vi "RT.vi"() -> ()   [LabVIEW 2012]
uses:
  Type/_RT Instrument State.ctl
  Type/RT Loop Events.ctl
  Type/_RT Parameter.ctl
  Type/_RT Active Ch.ctl
  Type/_RT Expt.ctl
  Type/_Run Mode.ctl
  Type/_RT Mass Range.ctl
  Type/_RT Res Type.ctl
  Type/_LED States.ctl
  Type/_LCD Line1 Msg.ctl
  Type/_LCD Line2 Msg.ctl
  Type/_RT LED Num.ctl
  Type/_Pump Parameter.ctl
  Type/_RW Status.ctl
  Type/_RT Serial Command.ctl
  Type/_FPGA Indicator.ctl
  _RT Global.vi
  <vilib>/FPGAPlugInAG/sbRIO-9602/niLvFpga_Open_sbRIO-9602.vi
  <vilib>/Utility/error.llb/Error Cluster From Error Code.vi
  <vilib>/rvi/errors/niLvFpgaAdjustHostInterfaceError.vi
  <vilib>/Utility/config.llb/Read Key (Boolean).vi
  <vilib>/Utility/config.llb/Read Key (String).vi
  <vilib>/Utility/config.llb/Write Key (Boolean).vi
  <vilib>/Utility/config.llb/Write Key (String).vi
  <vilib>/rvi/interface/nirviOpenFPGA/nirviOpenFPGA.xnode
  FPGA Bitfiles/FPGA9602.lvbitx
  <vilib>/rvi/interface/nirviMethod/nirviMethod.xnode
  <vilib>/rvi/interface/nirviReadWriteControl/nirviReadWriteControl.xnode
  <vilib>/Utility/config.llb/NI_LVConfig.lvlib
  <vilib>/NI_Real-Time Target Support.lvlib
  <vilib>/rvi/errors/niLvFpgaMergeErrorWithErrorCode.vi
  NiFpgaLv.dll
  <vilib>/FPGAPlugInAG/sbRIO-9602/niLvFpga_ConfigureFifo_sbRIO-9602.vi
  <vilib>/FPGAPlugInAG/sbRIO-9602/niLvFpga_StartFifo_sbRIO-9602.vi
panel:
  out "Disconnection#":u8
  out "Message Type":string
  out "Rt Loop Events":T1
  out "code":i32
  out "InstrState":T2=enum."Mass Spectrometer is Off"
  out "Fault":bool
  out "Ready":bool
  out "Running":bool
  out "RunMode":i32
  in  "RT Version":u32=900140920
  out "FPGA Version":u32
  out "Time (s)":dbl
  out "Connected?":bool
  # "Run  Status"
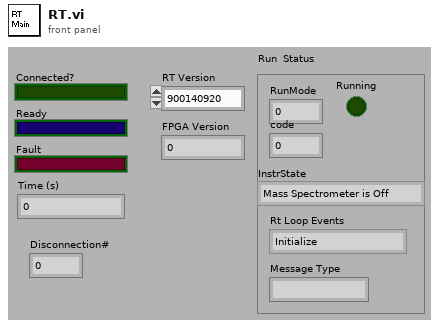
[diagram p1: front panel]
types:
  T1 = typedef "RT Loop Events.ctl" = enum16{"Initialize", "Wait for Connection", "Wait for Command", "Send Reply"}
  T2 = typedef "_RT Instrument State.ctl" = enum16{"Initializing", "Mass Spectrometer is Off", "Starting Up", "Turning Power Off", "Going to Standby", "Roughing Pump Ready", "Turning Turbo Off", "Turbo Startup", "Turbopump Ready", "Checking Vacuum", "Going to Ready", "Ready", "Running", "Source Standby", "Lost Communication", "Shutting Down", "Fault", "24V Standby", "Go to 24V Standby", "Turbopump Ready-Waiting"}
  T3 = typedef "_RT Parameter.ctl" = cluster{"RunMode":i32, "Initial Ch":T4[], "Sync":u8, "Expt":T5[], "EqTime(mS)":i32}
  T4 = typedef "_RT Active Ch.ctl" = cluster{"Start":i32, "Step":i32, "ChID":i32}
  T5 = typedef "_RT Expt.ctl" = cluster{"StartT(mS)":i32, "#Cycles":i32, "Scan Type":T6, "PauseT(uS)":i32, "Polarity":u8, "DelayT(mS)":i32, "Active Ch":T4[], "Mass Range":T7[]}
  T6 = typedef "_Run Mode.ctl" = enum16{"MRM (Q1/Q2)", "Q1 Scan", "Q1 SRM", "Q2 Scan", "Q2 SRM", "Product Scan", "Precursor Scan", "Neutral Loss", "Neutral Gain"}
  T7 = typedef "_RT Mass Range.ctl" = cluster{"Steps":i32, "Dwell(uS)":i32, "Resolution Type":T8, "Ramping Ch":T4[]}
  T8 = typedef "_RT Res Type.ctl" = u16
  T9 = typedef "Semaphore RefNum" = refnum<k1>
  T10 = typedef "_RT Instrument 2.ctl" = cluster{"Table":T11[], "Instrument":string[]}
  T11 = typedef "_RT Configuration 2.ctl" = cluster{"Name":string, "Ch#":u8, "Min":dbl, "Max":dbl, "Def+":dbl, "Def-":dbl, "Offset":dbl, "Slope":dbl, "Type":u8, "Description":string, "SettleT":dbl}
  T12 = cluster{"Rt Loop Events":T1, "Connection ID":refnum<k5>, "Parameter":T3, "Info":string, "Data Array":i32[], "error":errorcluster}
  T13 = typedef "_Pump Parameter.ctl" = enum16{"Turn Pump Motor On", "Turn Pump Motor Off", "Read Pump Oil Deficiency", "Read Rotation Switch Point Attained", "Read Ele. Drive Over Temperature", "Read Pump Over Temperature", "Read Set Rotation Speed Attained", "Read Turbopump Accelerates", "Read Actual Rotation Speed in Hz", "Read Motor Current in A", "Read Operating Hours in h", "Read Motor Voltage in V", "Read Motor Power in W", "Set Rotation Speed Switchpoint in %", "Clear Error", "Read Error Code", "Read Bearing Temperature", "Read Hardware Version", "Read Firmware Version", "Read Operating Hours (Drive)", "Read Rotational Speed (rpm)", "Read Power Stage Temperature", "Read Electronics Temperature", "Read Upper Pump Temperature", "Read Motor Temperature", "Read Error Code History, 1", "Read Error Code History, 2", "Read Error Code History, 3", "Read Error Code History, 4", "Read Error Code History, 5", "Read Error Code History, 6", "Read Error Code History, 7", "Read Error Code History, 8", "Read Error Code History, 9", "Read Error Code History, 10"}
  T14 = typedef "_RW Status.ctl" = enum8{"Done", "Do Read", "Do Write", "Set Latch1", "Set Latch2", "Set Latch3", "Set Latch4", "RP ON", "EL ON", "Serial Send", "Set LC Out", "Get LC In", "Read VAC", "Table Test", "Get Interlock", "Do Read2", "Do Write2"}
  T15 = typedef "_RT Serial Command.ctl" = cluster{"Port Type":u16, "baud rate (9600)":u32, "data bits (8)":u16, "stop bits (1)":u16, "parity (0:none)":u16, "DoRead":bool, "Command":string}
  T16 = typedef "_FPGA Indicator.ctl" = enum16{"Done", "Ready", "Count Available", "SendSerial", "LED State"}
  T17 = typedef "NI_LVConfig.lvlib/Config Data RefNum.ctl" = refnum<k1>
  T18 = typedef "_RT Startup Options.ctl" = cluster{"Door":bool, "Curtain":bool, "Pressure":bool, "Turbo":bool, "SysPoll":bool, "GasFlag":bool}
  T19 = cluster{"Info":string, "Data Array":i32[], "error":errorcluster}
  T20 = typedef "_RT LED Num.ctl" = enum8{"ReadKey", "ClearKeyBuffer", "ClearLCD", "BacklightOn"}
  T21 = typedef "_LED States.ctl" = enum8{"Idle", "Solid B", "Solid R", "Solid P", "Off B", "Off R", "Off P", "Off BRP", "Off RP", "Flash R&P", "Flash P"}
  T22 = typedef "_LCD Line2 Msg.ctl" = u16
  T23 = typedef "_LCD Line1 Msg.ctl" = u16
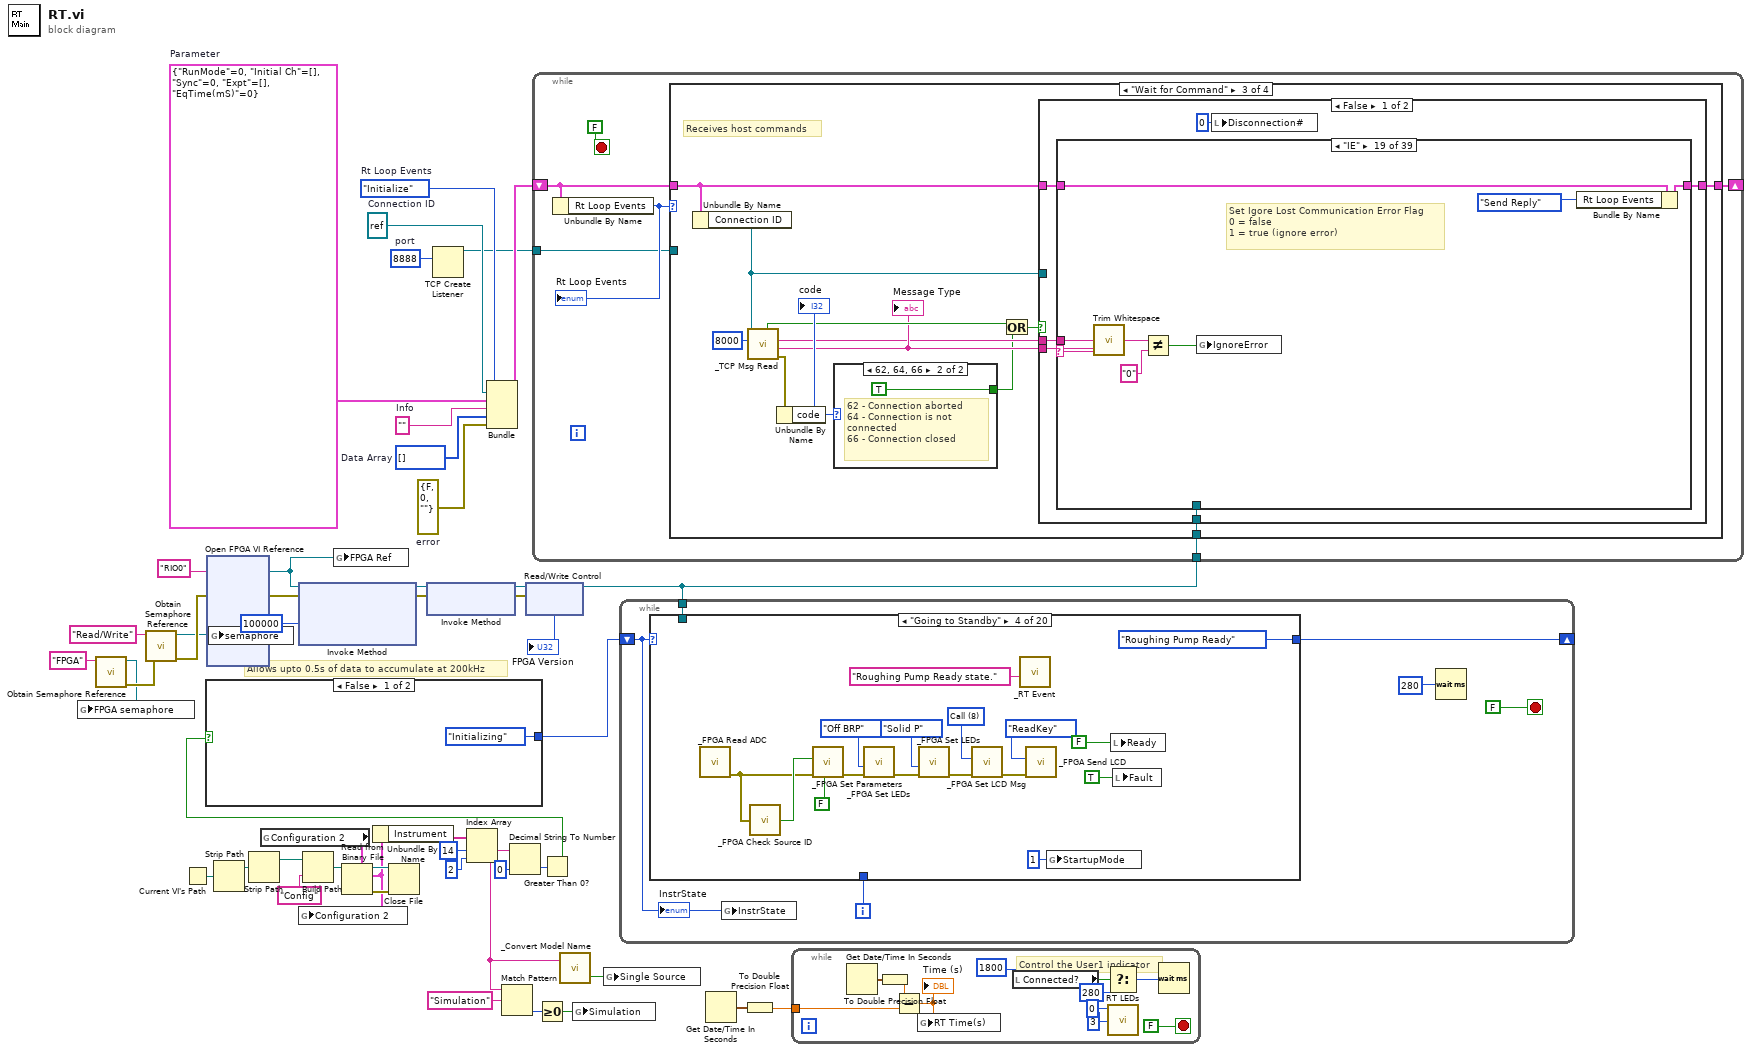
[diagram p0: block diagram]
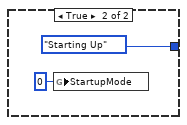
[diagram p2: hidden frame]
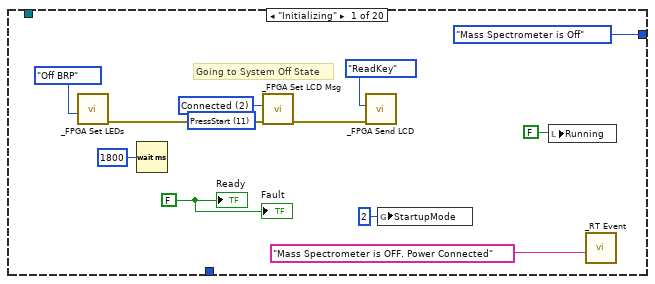
[diagram p3: hidden frame]
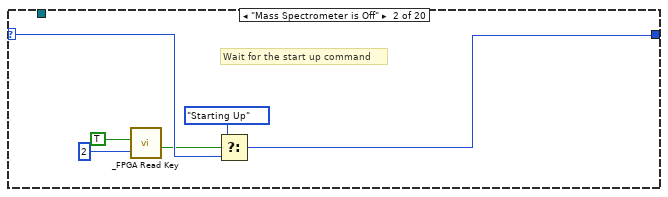
[diagram p4: hidden frame]
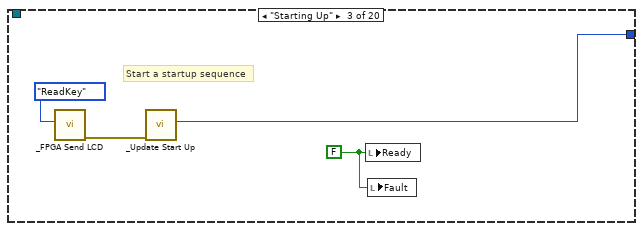
[diagram p5: hidden frame]
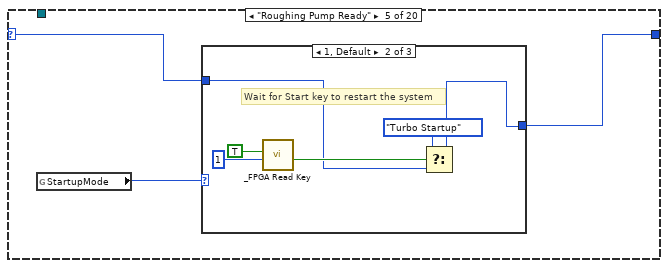
[diagram p6: hidden frame]
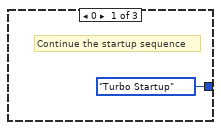
[diagram p7: hidden frame]
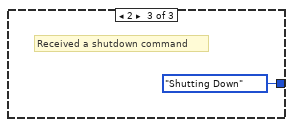
[diagram p8: hidden frame]
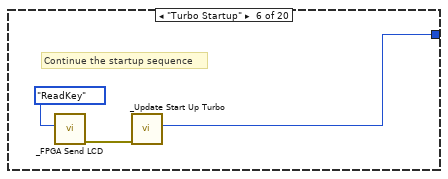
[diagram p9: hidden frame]
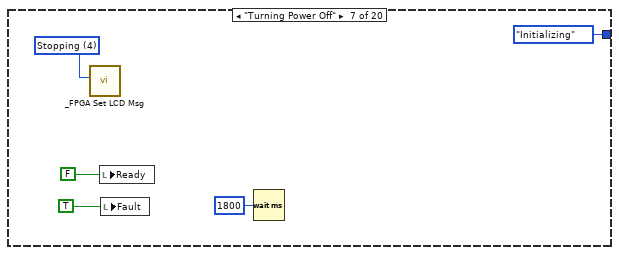
[diagram p10: hidden frame]
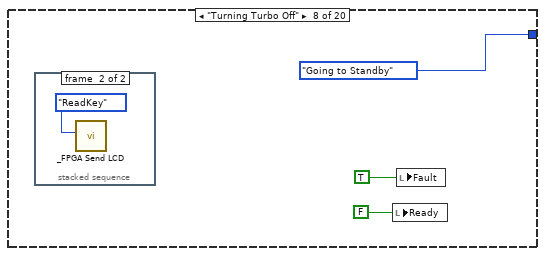
[diagram p11: hidden frame]
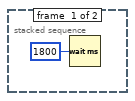
[diagram p12: hidden frame]
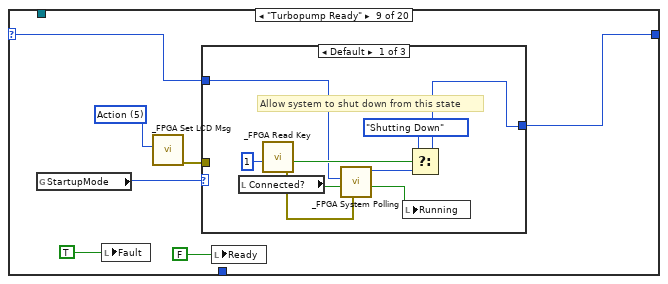
[diagram p13: hidden frame]
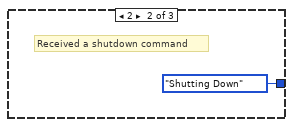
[diagram p14: hidden frame]
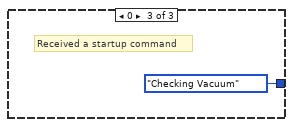
[diagram p15: hidden frame]
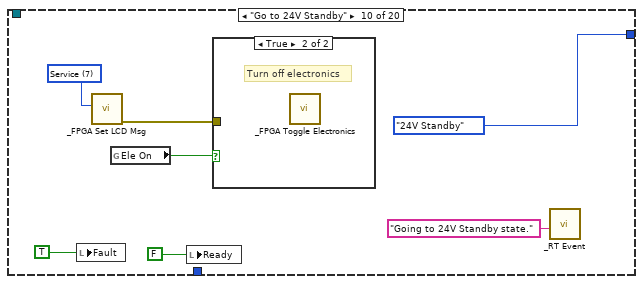
[diagram p16: hidden frame]
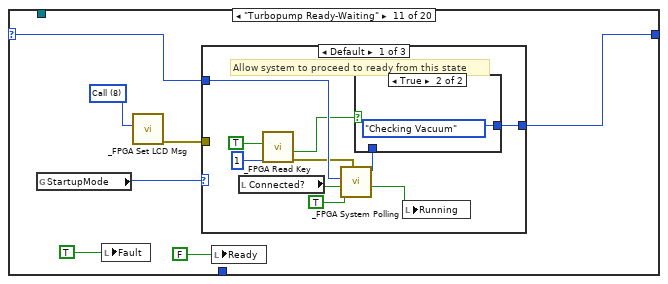
[diagram p18: hidden frame]
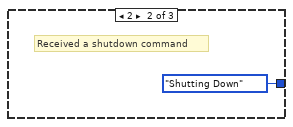
[diagram p20: hidden frame]
diagram:
  w34 = T3 {"RunMode"=0, "Initial Ch"=[], "Sync"=0, "Expt"=[], "EqTime(mS)"=0}  # Parameter
  w36 = u16 8888  # port
  w44 = i32[] []  # Data Array
  w45 = ""  # Info
  w46 = errorcluster {"status"=FALSE, "code"=0, "source"=""}  # error
  w48 = refnum<k5> refnum  # Connection ID
  w49 = RT_Loop_Events."Initialize"  # Rt Loop Events
  # "Allows upto 0.5s of data to accumulate at 200kHz"
  n1 = call <vilib>:"Obtain Semaphore Reference.vi"("name (unnamed)"="FPGA") -> ("error out"=w13:errorcluster, "semaphore"=w11:T9)  [unwired: 2 in, 3 out]
  n2 = global write "_RT Global.vi" "FPGA semaphore"(w11) -> ()
  n3 = call <vilib>:"Obtain Semaphore Reference.vi"("error in (no error)"=w13, "name (unnamed)"="Read/Write") -> ("error out"=w16:errorcluster, "semaphore"=w15:T9)  [unwired: 1 in, 3 out]
  n4 = Current VI's Path() -> (path=w31:path)
  n5 = xnode "Open FPGA VI Reference"("error in"=w16, "resource name"="RIO0") -> ("FPGA VI Reference Out"=w1:refnum<k20>, "error out"=w38:errorcluster)
  n6 = global write "_RT Global.vi" "semaphore"(w15) -> ()
  n7 = Strip Path(path=w31) -> (stripped path=w32:path)  [unwired: 1 out]
  n8 = Strip Path(path=w32) -> (stripped path=w25:path)  [unwired: 1 out]
  n9 = global read "_RT Global.vi" "Configuration 2"() -> (w28:T10)
  n10 = xnode "Invoke Method"("FPGA VI Reference In"=w1, "error in"=w38, "Requested Depth"=u32 100000 ("Depth")) -> ("FPGA VI Reference Out"=w40:refnum<k20>, "error out"=w41:errorcluster)  [unwired: 1 out]
  n11 = Build Path(base path=w25, name or relative path="Config" ("key")) -> (appended path=w30:path)
  n12 = global write "_RT Global.vi" "FPGA Ref"(w1) -> ()
  n13 = Read from Binary File(5:w28, 11:w30) -> (0:w27:errorcluster, 2:w24:T10, 3:w26:refnum<file>)  [unwired: 1 in, 4 out]
  n14 = global write "_RT Global.vi" "Configuration 2"(w24) -> ()
  n15 = Unbundle By Name(w24) -> ("Instrument"=w23:string[])
  n16 = Close File(refnum=w26, error in=w27) -> ()  [unwired: 2 out]
  n17 = xnode "Invoke Method"("FPGA VI Reference In"=w40, "error in"=w41) -> ("FPGA VI Reference Out"=w42:refnum<k20>, "error out"=w43:errorcluster)
  n18 = TCP Create Listener(10:w36) -> (3:w35:refnum<k5>)  [unwired: 1 in, 5 out]
  n19 = Index Array(array=w23, index #1=14 ("index"), index #2=2 ("index")) -> (element #1=w20:string, element #2=w6:string)
  n20 = Bundle("Rt Loop Events"=w49, "Connection ID"=w48, "Parameter"=w34, "Info"=w45, "Data Array"=w44, "error"=w46) -> (w47:T12)  [unwired: 1 out]
  n21 = Match Pattern(string=w6, regular expression="Simulation") -> (offset past match=w9:i32)  [unwired: 4 out]
  n22 = Decimal String To Number(string=w20, default (0L)=0 ("default (0 I32)")) -> (number=w19:i32)  [unwired: 2 out]
  n23 = xnode "Read/Write Control"("FPGA VI Reference In"=w42, "error in"=w43) -> ("FPGA VI Reference Out"=w4:refnum<k20>, "Version"=→"FPGA Version":u32)  [unwired: 1 out]
  n24 = while {
    shift-right: [w52] -> _
    shift-left: w47 -> [w53]
    tunnel: w4 -> [w51]
    tunnel: w35 -> [w50]
    stop <- FALSE stop-if-true
    n25 = Unbundle By Name(w53) -> ("Rt Loop Events"=w54:T1)
    "Rt Loop Events" <- w54
    n26 = case shown="\"Wait for Command\"" w54 {
      tunnel: w53 -> [w83 w124 w144 w782]
      tunnel: [w82 w123 w143 w781] -> w52
      tunnel: w51 -> [_ _ w139 _]
      tunnel: w50 -> [_ w121 _ _]
      frame "Initialize", Default {
        w56 = FALSE ("Connected?")
        w76 = FALSE ("Connected?")
        w69 = "RT" ("section")
        # "Initialize All Instrument Parameters"
        n27 = stacked-sequence {
          frame #0 {
            n28 = call "_Read RT Table.vi"("key"="Cal") -> ("Table"=w85:dbl[][])  [unwired: 2 in, 4 out]
            n29 = global write "_RT Global.vi" "Q1 Cal"(w85) -> ()
            n30 = call "_Read RT Table.vi"("key"="Cal2") -> ("Table"=w86:dbl[][])  [unwired: 2 in, 4 out]
            n31 = global write "_RT Global.vi" "Q2 Cal"(w86) -> ()
            n32 = call "_Read RT Table.vi"("key"="Cal3") -> ("Table"=w87:dbl[][])  [unwired: 2 in, 4 out]
            n33 = global write "_RT Global.vi" "Q1 -Cal"(w87) -> ()
            n34 = call "_Read RT Table.vi"("key"="Cal4") -> ("Table"=w88:dbl[][])  [unwired: 2 in, 4 out]
            n35 = global write "_RT Global.vi" "Q2 -Cal"(w88) -> ()
            n36 = call "_Read RT Table.vi"("key"="Res") -> ("Table"=w89:dbl[][])  [unwired: 2 in, 4 out]
            n37 = global write "_RT Global.vi" "Q1 Res Hi"(w89) -> ()
            n38 = call "_Read RT Table.vi"("key"="Res2") -> ("Table"=w90:dbl[][])  [unwired: 2 in, 4 out]
            n39 = global write "_RT Global.vi" "Q2 Res Hi"(w90) -> ()
            n40 = call "_Read RT Table.vi"("key"="Res3") -> ("Table"=w91:dbl[][])  [unwired: 2 in, 4 out]
            n41 = global write "_RT Global.vi" "Q1 Res Med"(w91) -> ()
            n42 = call "_Read RT Table.vi"("key"="Res4") -> ("Table"=w92:dbl[][])  [unwired: 2 in, 4 out]
            n43 = global write "_RT Global.vi" "Q2 Res Med"(w92) -> ()
            n44 = call "_Read RT Table.vi"("key"="Res5") -> ("Table"=w93:dbl[][])  [unwired: 2 in, 4 out]
            n45 = global write "_RT Global.vi" "Q1 Res Lo"(w93) -> ()
            n46 = call "_Read RT Table.vi"("key"="Res6") -> ("Table"=w94:dbl[][])  [unwired: 2 in, 4 out]
            n47 = global write "_RT Global.vi" "Q2 Res Lo"(w94) -> ()
            n48 = call "_Read RT Table.vi"("key"="Res7") -> ("Table"=w95:dbl[][])  [unwired: 2 in, 4 out]
            n49 = global write "_RT Global.vi" "Q1 -Res Hi"(w95) -> ()
            n50 = call "_Read RT Table.vi"("key"="Res8") -> ("Table"=w96:dbl[][])  [unwired: 2 in, 4 out]
            n51 = global write "_RT Global.vi" "Q2 -Res Hi"(w96) -> ()
            n52 = call "_Read RT Table.vi"("key"="Res9") -> ("Table"=w97:dbl[][])  [unwired: 2 in, 4 out]
            n53 = global write "_RT Global.vi" "Q1 -Res Med"(w97) -> ()
            n54 = call "_Read RT Table.vi"("key"="Res10") -> ("Table"=w98:dbl[][])  [unwired: 2 in, 4 out]
            n55 = global write "_RT Global.vi" "Q2 -Res Med"(w98) -> ()
            n56 = call "_Read RT Table.vi"("key"="Res11") -> ("Table"=w99:dbl[][])  [unwired: 2 in, 4 out]
            n57 = global write "_RT Global.vi" "Q1 -Res Lo"(w99) -> ()
            n58 = call "_Read RT Table.vi"("key"="Res12") -> ("Table"=w100:dbl[][])  [unwired: 2 in, 4 out]
            n59 = global write "_RT Global.vi" "Q2 -Res Lo"(w100) -> ()
          }
          frame #1 {
            n60 = for {
              N: 16 -> [_]
              i -> [w118]
              n61 = call "_Update Cal or Res Data.vi"("Table Type"=w118) -> ()  [unwired: 2 in, 5 out]
            }
          }
        }
        n62 = Current VI's Path() -> (path=w73:path)
        n63 = Strip Path(path=w73) -> (stripped path=w74:path)  [unwired: 1 out]
        n64 = Strip Path(path=w74) -> (stripped path=w58:path)  [unwired: 1 out]
        n65 = global read "_RT Global.vi" "ADC Table"() -> (w60:T11[])
        n66 = Build Path(base path=w58, name or relative path="ADC" ("key")) -> (appended path=w59:path)
        n67 = Read from Binary File(5:w60, 11:w59) -> (0:w62:errorcluster, 2:w61:T11[], 3:w63:refnum<file>)  [unwired: 1 in, 4 out]
        n68 = global write "_RT Global.vi" "ADC Table"(w61) -> ()
        n69 = Close File(refnum=w63, error in=w62) -> ()  [unwired: 2 out]
        n70 = Bundle By Name(cluster=w83, "Rt Loop Events"=RT_Loop_Events."Wait for Connection") -> (w82:T12)
        n71 = call "_RT Open Preference File.vi"() -> ("refnum"=w75:T17)  [unwired: 7 out]
        n72 = global read "_RT Global.vi" "StartupOptions"() -> (w64:T18)
        n73 = local write "Connected?"(w56) -> ()
        n74 = local write "Ready"(w56) -> ()
        n75 = call-poly <vilib>:"Read Key.vi"("section"=w69, "default value"=w76, "key"="Q1Pol", "refnum"=w75) -> ("value"=w77:bool, "refnum out"=w78:T17)  [unwired: 1 in, 5 out]
        n76 = local write "Fault"(w56) -> ()
        n77 = global write "_RT Global.vi" "IgnoreError"(w56) -> ()
        n78 = global write "_RT Global.vi" "Ele On"(w56) -> ()
        n79 = Flatten To String(anything=w64) -> (data string=w67:string)  [unwired: 1 in, 4 out]
        n80 = call-poly <vilib>:"Read Key.vi"("section"=w69, "default value"=w76, "key"="Q2Pol", "refnum"=w78) -> ("value"=w72:bool, "refnum out"=w71:T17)  [unwired: 1 in, 5 out]
        n81 = global write "_RT Global.vi" "Q2 POL"(w72) -> ()
        n82 = global write "_RT Global.vi" "Q1 POL"(w77) -> ()
        n83 = call-poly <vilib>:"Read Key.vi"("section"=w69, "default value"=w67, "key"="SUOpt", "refnum"=w71) -> ("value"=w66:string, "refnum out"=w68:T17)  [unwired: 2 in, 4 out]
        n84 = Unflatten From String(type=w64, binary string=w66) -> (value=w65:T18)  [unwired: 1 in, 4 out]
        n85 = global write "_RT Global.vi" "StartupOptions"(w65) -> ()
        n86 = call <vilib>:"Close Config Data.vi"("write file if changed (T)"=TRUE ("write configuration file? (T)"), "refnum"=w68) -> ()  [unwired: 1 in, 9 out]
      }
      frame "Wait for Connection" {
        # "Waits for new host connection"
        n87 = TCP Wait On Listener(9:-1 ("timeout ms (wait forever: -1)"), 11:w121) -> (0:w122:errorcluster, 4:w120:refnum<k5>)  [unwired: 1 in, 4 out]
        n88 = case shown="No Error" w122 {
          tunnel: w124 -> [w131 w134]
          tunnel: w120 -> [w128 _]
          tunnel: [w130 w132] -> w123
          frame No Error {
            n89 = local write "Disconnection#"(u8 0 ("Disconnection#")) -> ()
            n90 = local write "Connected?"(TRUE ("Connected?")) -> ()
            n91 = call "_RT Event.vi"("Event"="PC Communication Established") -> ()  [unwired: 2 in, 5 out]
            n92 = Bundle By Name(cluster=w131, "Connection ID"=w128, "Rt Loop Events"=RT_Loop_Events."Wait for Command") -> (w130:T12)
          }
          frame Error {
            n93 = Bundle By Name(cluster=w134, "Rt Loop Events"=RT_Loop_Events."Wait for Connection") -> (w132:T12)
          }
        }
      }
      frame "Wait for Command" {
        # "Receives host commands"
        n94 = Unbundle By Name(w144) -> ("Connection ID"=w136:refnum<k5>)
        n95 = call "_TCP Msg Read.vi"("timeout ms (10000)"=8000 ("millisecond multiple"), "connection ID"=w136) -> ("error out"=w138:errorcluster, "Message Type"=w142:string, "Data Stream"=w141:string, "Timed Out?"=w145:bool)  [unwired: 3 in, 3 out]
        "Message Type" <- w142
        n96 = Unbundle By Name(w138) -> ("code"=w146:i32)
        "code" <- w146
        n97 = case shown="62, 64, 66" w146 {
          tunnel: [_ TRUE ("abort (F)")] -> w135
          frame Default {
          }
          frame 62, 64, 66 {
            # "62 - Connection aborted\n64 - Connection is not connected\n66 - Connection closed"
          }
        }
        n98 = Or(x=w145, y=w135) -> (x .or. y?=w137:bool)
        n99 = case shown="False" w137 {
          tunnel: w144 -> [w151 w767]
          tunnel: [w150 w766] -> w143
          tunnel: w142 -> [w148 _]
          tunnel: w141 -> [w152 _]
          tunnel: w139 -> [w149 _]
          tunnel: w136 -> [_ w763]
          frame False {
            n100 = case shown="\"IE\"" w148 {
              selector: w148 -> [_ _ _ _ _ _ _ _ _ _ _ _ _ _ _ _ _ _ _ _ _ _ _ _ _ _ _ _ _ _ _ _ _ _ _ _ _ _ w759]
              tunnel: w152 -> [_ w172 w177 w190 w222 w231 w253 w273 _ w293 _ _ _ _ _ w361 _ w426 w450 w459 _ w465 w483 w491 w499 _ w508 w532 w547 _ w579 w582 w592 w612 w632 w648 w695 w709 _]
              tunnel: w151 -> [w157 w169 w182 w207 w225 w234 w250 w270 w287 w295 w301 w306 w315 w350 w358 w365 w423 w430 w453 w456 w463 w475 w480 w488 w496 w506 w513 w535 w545 w557 w576 w586 w599 w610 w630 w645 w705 w715 w755]
              tunnel: [w156 w168 w181 w206 w224 w233 w249 w269 w286 w294 w300 w305 w314 w349 w357 w364 w422 w429 w452 w455 w462 w474 w479 w487 w495 w505 w512 w534 w544 w556 w575 w585 w598 w609 w629 w644 w704 w712 w754] -> w150
              tunnel: w149 -> [_ _ _ _ _ _ _ _ _ _ _ _ w307 w346 _ _ w419 _ _ _ _ _ _ _ _ _ _ _ w543 _ _ _ w597 w608 w628 w641 w694 _ _]
              frame "AG" {
                # "Get ADC Table"
                n101 = global read "_RT Global.vi" "ADC Table"() -> (w154:T11[])
                n102 = Flatten To String(anything=w154) -> (data string=w153:string)  [unwired: 1 in, 4 out]
                n103 = Bundle By Name(cluster=w157, "Rt Loop Events"=RT_Loop_Events."Send Reply", "Info"=w153) -> (w156:T12)
              }
              frame "AS" {
                # "Set ADC Table"
                n104 = global read "_RT Global.vi" "ADC Table"() -> (w171:T11[])
                n105 = Unflatten From String(type=w171, binary string=w172) -> (value=w162:T11[], error out=w159:errorcluster)  [unwired: 1 in, 3 out]
                n106 = Current VI's Path() -> (path=w165:path)
                n107 = Strip Path(path=w165) -> (stripped path=w166:path)  [unwired: 1 out]
                n108 = Strip Path(path=w166) -> (stripped path=w167:path)  [unwired: 1 out]
                n109 = Build Path(base path=w167, name or relative path="ADC" ("key")) -> (appended path=w163:path)
                n110 = global write "_RT Global.vi" "ADC Table"(w162) -> ()
                n111 = Write to Binary File(file (use dialog)=w163, data=w162, error in=w159) -> (refnum out=w160:refnum<file>, error out=w161:errorcluster)  [unwired: 4 out]
                n112 = Close File(refnum=w160, error in=w161) -> (error out=w158:errorcluster)  [unwired: 1 out]
                n113 = Bundle By Name(cluster=w169, "Rt Loop Events"=RT_Loop_Events."Send Reply", "error"=w158) -> (w168:T12)
              }
              frame "AU" {
                # "Send auxiliary update command"
                n114 = Scan From String(format string="%d,%f", input string=w177, default 1=-1 ("default value 1"), default 2=sgl 0.0 ("default value 2")) -> (output 1=w176:i32, output 2=w175:sgl)  [unwired: 2 in, 3 out]
                n115 = call "_FPGA Auxiliary Update.vi"("Setting Value"=w175, "Command Type"=w176) -> ("error out"=w174:errorcluster, "Return Value"=w173:string)  [unwired: 1 in, 3 out]
                n116 = Bundle By Name(cluster=w182, "Rt Loop Events"=RT_Loop_Events."Send Reply", "Info"=w173, "error"=w174) -> (w181:T12)
              }
              frame "BS" {
                # "Get Brief Instrument Status Report"
                n117 = local read "Running"() -> (w184:bool)
                n118 = Empty String/Path?(string/path=w190) -> (empty?=w189:bool)
                n119 = global read "_RT Global.vi" "ADC Values"() -> (w187:i32[])
                n120 = call "_Calculate ADC Value.vi"("ADC Values"=w187, "ADC Channel (64)"=u8 64) -> ("User Value"=w195:sgl, "In Range?"=w186:bool)  [unwired: 1 out]
                n121 = call "_Calculate ADC Value.vi"("ADC Values"=w187, "ADC Channel (64)"=u8 72) -> ("In Range?"=w185:bool)  [unwired: 2 out]
                n122 = for {
                  tunnel: i32[] [119, 113, 114, 110, 108, 105, 120, 72, 71, 65, 67, 66, 68, 106, 107, 109] -> [w216] mode=indexing
                  tunnel: w187 -> [w217]
                  tunnel: [w215] -> w202 mode=indexing
                  tunnel: [w214] -> w204 mode=indexing
                  n123 = call "_Calculate ADC Value.vi"("ADC Values"=w217, "ADC Channel (64)"=w216) -> ("User Value"=w215:sgl, "In Range?"=w214:bool)  [unwired: 1 out]
                }
                n124 = case shown="False" w184 {
                  tunnel: [w209 830 ("Speed")] -> w197
                  frame False {
                    n125 = call "_FPGA Turbo Control.vi"("Command"=_Pump_Parameter."Read Actual Rotation Speed in Hz") -> ("Speed"=w209:i32)  [unwired: 3 in, 5 out]
                  }
                  frame True {
                  }
                }
                n126 = Build Array (concatenate)(w202, w195, w197) -> (w198:sgl[])
                n127 = Greater Or Equal?(x=w197, y=830) -> (x >= y?=w199:bool)
                n128 = Build Array (concatenate)(w204, w186, w199, w185) -> (w200:bool[])
                n129 = Flatten To String(anything=w198) -> (data string=w192:string)  [unwired: 1 in, 4 out]
                n130 = case shown="True" w189 {
                  tunnel: [_ w212] -> w194
                  frame False {
                    # "for Server"
                  }
                  frame True {
                    # "Ion Sniffer"
                    n131 = call "_RT Event.vi"("Action (Write)"=enum16{"Write", "Read"}."Read") -> ("Log"=w212:string)  [unwired: 2 in, 4 out]
                  }
                }
                n132 = Boolean To (0,1)(Boolean=w200) -> (0, 1=w203:i16[])
                n133 = Format Into String(format string="%s<RTLog>%s", w192, w194) -> (resulting string=w191:string)  [unwired: 2 in, 1 out]
                n134 = Bundle By Name(cluster=w207, "Rt Loop Events"=RT_Loop_Events."Send Reply", "Data Array"=w203, "Info"=w191) -> (w206:T12)
              }
              frame "CC" {
                # "Set contact closure output logics:\n0 for Shimadzu; 1 for others"
                n135 = Type Cast(type=u16 0, x=w222) -> (*(type *) &x=w219:u16)
                n136 = call "_FPGA Write Data.vi"("Write Mode (Do Write)"=_RW_Status."Do Write", "Data"=w219, "Address"=u16 399) -> ("error out"=w218:errorcluster)  [unwired: 3 in, 2 out]
                n137 = Bundle By Name(cluster=w225, "Rt Loop Events"=RT_Loop_Events."Send Reply", "error"=w218) -> (w224:T12)
              }
              frame "CI" {
                # "Set contact closure input logics:\nOption    LC1        LC2\n     0        High      High\n     1        Low        High\n     2        High       Low\n     3        Low        Low"
                n138 = Type Cast(type=u16 0, x=w231) -> (*(type *) &x=w228:u16)
                n139 = call "_FPGA Write Data.vi"("Write Mode (Do Write)"=_RW_Status."Do Write", "Data"=w228, "Address"=u16 409) -> ("error out"=w227:errorcluster)  [unwired: 3 in, 2 out]
                n140 = Bundle By Name(cluster=w234, "Rt Loop Events"=RT_Loop_Events."Send Reply", "error"=w227) -> (w233:T12)
              }
              frame "CP" {
                # "Set Source Polarity:"
                # "Set CEM POL for Latch4"
                # "Set S1 POL, S2 POL for Latch3"
                # "Set COR POL, CUR POL for Latch2"
                n141 = Type Cast(type=u16 0, x=w253) -> (*(type *) &x=w238:u16)
                n142 = Greater Than 0?(x=w238) -> (x > 0?=w237:bool)
                n143 = Number To Boolean Array(number=u16 0) -> (Boolean array=w242:bool[])
                n144 = Replace Array Subset(array=w242, new element #1=w237, index #1=0 ("index"), new element #2=w237, index #2=1 ("index")) -> (w239:bool[])
                n145 = Boolean Array To Number(Boolean array=w239) -> (number=w236:u16)
                n146 = call "_FPGA Set Digi Line.vi"("States"=w236, "Line (Set Latch1)"=_RW_Status."Set Latch2" ("Write Mode (Do Write)")) -> ("error out"=w247:errorcluster)  [unwired: 2 in, 3 out]
                n147 = call "_FPGA Set Digi Line.vi"("error in"=w247, "States"=w236, "Line (Set Latch1)"=_RW_Status."Set Latch3" ("Write Mode (Do Write)")) -> ("error out"=w245:errorcluster)  [unwired: 1 in, 3 out]
                n148 = call "_FPGA Set Digi Line.vi"("error in"=w245, "States"=w236, "Line (Set Latch1)"=_RW_Status."Set Latch4" ("Write Mode (Do Write)")) -> ("error out"=w244:errorcluster)  [unwired: 1 in, 3 out]
                n149 = Bundle By Name(cluster=w250, "Rt Loop Events"=RT_Loop_Events."Send Reply", "error"=w244) -> (w249:T12)
              }
              frame "DP" {
                w258 = "RT" ("section")
                # "Set Q1 POL, Q2 POL, Q1DC EN, Q2DC EN"
                n150 = Type Cast(type=u16 0, x=w273) -> (*(type *) &x=w267:u16)
                n151 = Number To Boolean Array(number=w267) -> (Boolean array=w266:bool[])
                n152 = call "_FPGA Set Digi Line.vi"("States"=w267, "Line (Set Latch1)"=_RW_Status."Set Latch1" ("Write Mode (Do Write)")) -> ("error out"=w268:errorcluster)  [unwired: 2 in, 3 out]
                n153 = Index Array(array=w266) -> (element #1=w256:bool, element #2=w255:bool)  [unwired: 2 in]
                n154 = global write "_RT Global.vi" "Q1 POL"(w256) -> ()
                n155 = global write "_RT Global.vi" "Q2 POL"(w255) -> ()
                n156 = call "_RT Open Preference File.vi"() -> ("error"=w263:errorcluster, "refnum"=w262:T17)  [unwired: 6 out]
                n157 = call-poly <vilib>:"Write Key.vi"("section"=w258, "error in (no error)"=w263, "value"=w256, "key"="Q1Pol", "refnum"=w262) -> ("error out"=w260:errorcluster, "refnum out"=w259:T17)  [unwired: 5 out]
                n158 = call-poly <vilib>:"Write Key.vi"("section"=w258, "error in (no error)"=w260, "value"=w255, "key"="Q2Pol", "refnum"=w259) -> ("error out"=w265:errorcluster, "refnum out"=w264:T17)  [unwired: 5 out]
                n159 = call <vilib>:"Close Config Data.vi"("error in (no error)"=w265, "refnum"=w264) -> ()  [unwired: 1 in, 9 out]
                n160 = Bundle By Name(cluster=w270, "Rt Loop Events"=RT_Loop_Events."Send Reply", "error"=w268) -> (w269:T12)
              }
              frame "DS" {
                # "Get Detailed Instrument Status Report"
                n161 = local read "Running"() -> (w281:bool)
                n162 = local read "Ready"() -> (w282:bool)
                n163 = local read "Fault"() -> (w278:bool)
                n164 = Select(t="1", s=w281, f="0") -> (s? t:f=w283:string)
                n165 = Select(t=w283, s=w282, f="2") -> (s? t:f=w284:string)
                n166 = Select(t="3", s=w278, f=w284) -> (s? t:f=w277:string)
                n167 = call "_FPGA Get System Status.vi"("Server State"=w277) -> ("Status"=w285:string)  [unwired: 1 in, 5 out]
                n168 = Bundle By Name(cluster=w287, "Rt Loop Events"=RT_Loop_Events."Send Reply", "Info"=w285) -> (w286:T12)
              }
              frame "EL" {
                # "Toggle Electrics"
                n169 = Not Equal?(x=w293, y="0") -> (x != y?=w291:bool)
                n170 = Boolean To (0,1)(Boolean=w291) -> (0, 1=w290:i16)
                n171 = call "_FPGA Toggle Electronics.vi"("Ele On (1 for ON and 0 for OFF)"=w290) -> ("error out"=w289:errorcluster)  [unwired: 2 in, 5 out]
                n172 = Bundle By Name(cluster=w295, "Rt Loop Events"=RT_Loop_Events."Send Reply", "error"=w289) -> (w294:T12)
              }
              frame "EN" {
                w298 = u16 0 ("Address")
                # "End a Run"
                n173 = call "_FPGA Write Data.vi"("Data"=w298, "Address"=w298) -> ("error out"=w297:errorcluster)  [unwired: 4 in, 2 out]
                n174 = Bundle By Name(cluster=w301, "Rt Loop Events"=RT_Loop_Events."Send Reply", "error"=w297) -> (w300:T12)
              }
              frame "GC" {
                # "Get Configuration"
                n175 = global read "_RT Global.vi" "Configuration 2"() -> (w303:T10)
                n176 = Flatten To String(anything=w303) -> (data string=w302:string)  [unwired: 1 in, 4 out]
                n177 = Bundle By Name(cluster=w306, "Rt Loop Events"=RT_Loop_Events."Send Reply", "Info"=w302) -> (w305:T12)
              }
              frame "GD" {
                # "Get data and check for FPGA status"
                n178 = xnode "Read/Write Control"("FPGA VI Reference In"=w307) -> ("error out"=w309:errorcluster, "Running"=w312:bool)  [unwired: 1 in, 1 out]
                n179 = local write "Running"(w312) -> ()
                n180 = case shown="No Error" w309 {
                  selector: w309 -> [w317 w323]
                  tunnel: [w319 _] -> w310
                  tunnel: [w318 _] -> w311
                  tunnel: [w316 w321] -> w308
                  frame No Error {
                    n181 = call "_FPGA Read Counter.vi"("error in (no error)"=w317) -> ("error out"=w316:errorcluster, "size(s)"=w320:u32, "Data"=w318:i32[])  [unwired: 1 in, 1 out]
                    n182 = Number To Decimal String(number=w320) -> (decimal integer string=w319:string)  [unwired: 1 out]
                  }
                  frame Error {
                    n183 = call "_Construct Error Cluster.vi"("error in"=w323, "reason"="Engine Error:\nFound while getting data and checking FPGA status.") -> ("error out"=w321:errorcluster)  [unwired: 2 in, 3 out]
                  }
                }
                n184 = Bundle By Name(cluster=w315, "Rt Loop Events"=RT_Loop_Events."Send Reply", "Info"=w310, "Data Array"=w311, "error"=w308) -> (w314:T12)
              }
              frame "GI" {
                w337 = u32 60 ("y")
                # "Get Info"
                n185 = local read "Time (s)"() -> (w333:dbl)
                n186 = xnode "Read/Write Control"("FPGA VI Reference In"=w346) -> ("FPGA VI Reference Out"=w343:refnum<k20>, "error out"=w344:errorcluster, "Version"=w345:u32)  [unwired: 1 in]
                n187 = local read "Ready"() -> (w330:bool)
                n188 = xnode "Read/Write Control"("FPGA VI Reference In"=w343, "error in"=w344) -> ("Running"=w331:bool)  [unwired: 2 out]
                n189 = local write "Running"(w331) -> ()
                n190 = Select(t="System is running", s=w331, f="System is idling") -> (s? t:f=w328:string)
                n191 = To Unsigned Long Integer(number=w333) -> (unsigned 32bit integer=w335:u32)
                n192 = local read "Fault"() -> (w326:bool)
                n193 = Quotient & Remainder(x=w335, y=w337) -> (x-y*floor(x/y)=w338:u32, floor(x/y)=w336:u32)
                n194 = Select(t=w328, s=w330, f="System is not ready.") -> (s? t:f=w325:string)
                n195 = Select(t="System is in a fault state.", s=w326, f=w325) -> (s? t:f=w324:string)
                n196 = Quotient & Remainder(x=w336, y=w337) -> (x-y*floor(x/y)=w339:u32, floor(x/y)=w340:u32)
                n197 = Format Into String(format string="Ionica Firmware; FPGA: %d; RT: %d\n(%s: %dh%dm%ds)", w345, "RT Version", w324, w340, w339, w338) -> (resulting string=w347:string)  [unwired: 2 in, 1 out]
                n198 = Bundle By Name(cluster=w350, "Rt Loop Events"=RT_Loop_Events."Send Reply", "Info"=w347) -> (w349:T12)
              }
              frame "GL" {
                # "Get LC Inputs"
                n199 = call "_FPGA Read Data.vi"("Read Mode (Do Read)"=_RW_Status."Get LC In" ("R/W Status")) -> ("error out"=w351:errorcluster, "Data"=w352:u32)  [unwired: 4 in, 1 out]
                n200 = Split Number(x=w352) -> (hi(x)=w356:u16, lo(x)=w355:u16)
                n201 = Build Array(w356, w355) -> (w354:u16[])
                n202 = Bundle By Name(cluster=w358, "Rt Loop Events"=RT_Loop_Events."Send Reply", "Data Array"=w354, "error"=w351) -> (w357:T12)
              }
              frame "GP" {
                n203 = Decimal String To Number(string=w361) -> (number=w360:i32)  [unwired: 3 out]
                n204 = case shown="0" w360 {
                  selector: w360 -> [_ w372]
                  tunnel: [w366 w368] -> w362
                  frame 0 {
                    # "Get Parameter"
                    n205 = call "_Get FPGA Info.vi"() -> ("Info"=w366:string)  [unwired: 2 in, 5 out]
                  }
                  frame 1, Default {
                    # "Get Cal/Res Table"
                    n206 = Decrement(x=w372) -> (x-1=w371:i32)
                    n207 = case shown="13" w371 {
                      tunnel: [u16 500 ("Addr Offset") u16 550 ("Addr Offset") u16 600 ("Addr Offset") u16 650 ("Addr Offset") u16 700 ("Addr Offset") u16 750 ("Addr Offset") u16 800 ("Addr Offset") u16 850 ("Addr Offset") u16 900 ("Addr Offset") u16 950 ("Addr Offset") u16 1000 ("Addr Offset") u16 1050 ("Addr Offset") u16 1100 ("Addr Offset") u16 1150 ("Addr Offset") u16 1200 ("Addr Offset") u16 1250 ("Addr Offset")] -> w369
                      frame 0, Default {
                      }
                      frame 1 {
                      }
                      frame 2 {
                      }
                      frame 3 {
                      }
                      frame 4 {
                      }
                      frame 5 {
                      }
                      frame 6 {
                      }
                      frame 7 {
                      }
                      frame 8 {
                      }
                      frame 9 {
                      }
                      frame 10 {
                      }
                      frame 11 {
                      }
                      frame 12 {
                      }
                      frame 13 {
                      }
                      frame 14 {
                      }
                      frame 15 {
                      }
                    }
                    n208 = for {
                      N: 25 -> [_]
                      shift-right: [w378] -> w368
                      shift-left: "" -> [w381]
                      tunnel: w369 -> [w385]
                      shift-right: [w382] -> _
                      shift-left: _ -> [w383]
                      i -> [w388]
                      # "For each row"
                      n209 = Multiply(x=w388, y=2) -> (x*y=w386:i32)
                      n210 = Add(x=w386, y=w385) -> (x+y=w380:i32)
                      n211 = call "_FPGA Read Data.vi"("error in"=w383, "Address"=w380) -> ("error out"=w384:errorcluster, "Data"=w379:u32)  [unwired: 3 in, 1 out]
                      n212 = Increment(x=w380) -> (x+1=w376:i32)
                      n213 = call "_Format Memory Map String.vi"("User value"="Mass Value", "Data"=w379, "Address"=w380, "String In"=w381) -> ("String Out"=w377:string)  [unwired: 3 out]
                      n214 = call "_FPGA Read Data.vi"("error in"=w384, "Address"=w376) -> ("error out"=w382:errorcluster, "Data"=w375:u32)  [unwired: 3 in, 1 out]
                      n215 = call "_Format Memory Map String.vi"("User value"="DAC Value", "Data"=w375, "Address"=w376, "String In"=w377) -> ("String Out"=w378:string)  [unwired: 3 out]
                    }
                  }
                }
                n216 = Bundle By Name(cluster=w365, "Rt Loop Events"=RT_Loop_Events."Send Reply", "Info"=w362) -> (w364:T12)
              }
              frame "GS" {
                # "Get Status"
                n217 = xnode "Read/Write Control"("FPGA VI Reference In"=w419) -> ("Running"=w418:bool)  [unwired: 1 in, 2 out]
                n218 = local read "Ready"() -> (w417:bool)
                n219 = local write "Running"(w418) -> ()
                n220 = global read "_RT Global.vi" "InstrState"() -> (w407:T2)
                n221 = Select(t="1: The system is running", s=w418, f="0: The system is idling") -> (s? t:f=w414:string)
                n222 = local read "Fault"() -> (w415:bool)
                n223 = Select(t=w414, s=w417, f="2: The system is not ready") -> (s? t:f=w413:string)
                n224 = To Long Integer(number=w407) -> (32bit integer=w412:i32)
                n225 = Build Array(w412) -> (w411:i32[])
                n226 = Select(t="3: The system is in a fault state", s=w415, f=w413) -> (s? t:f=w408:string)
                n227 = Format Into String(format string="%s.  Instr State = %s.", w408, w407) -> (resulting string=w405:string)  [unwired: 2 in, 1 out]
                n228 = Bundle By Name(cluster=w423, "Rt Loop Events"=RT_Loop_Events."Send Reply", "Info"=w405, "Data Array"=w411) -> (w422:T12)
              }
              frame "GT" {
                # "Get a Calibration/Resolution Table"
                n229 = Decimal String To Number(string=w426) -> (number=w425:i32)  [unwired: 3 out]
                n230 = case shown="0, Default" w425 {
                  tunnel: [w431 w432 w433 w434 w435 w436 w437 w438 w439 w440 w441 w442 w443 w444 w445 w446] -> w424
                  frame 0, Default {
                    n231 = global read "_RT Global.vi" "Q1 Cal"() -> (w431:dbl[][])
                  }
                  frame 1 {
                    n232 = global read "_RT Global.vi" "Q2 Cal"() -> (w432:dbl[][])
                  }
                  frame 2 {
                    n233 = global read "_RT Global.vi" "Q1 -Cal"() -> (w433:dbl[][])
                  }
                  frame 3 {
                    n234 = global read "_RT Global.vi" "Q2 -Cal"() -> (w434:dbl[][])
                  }
                  frame 4 {
                    n235 = global read "_RT Global.vi" "Q1 Res Hi"() -> (w435:dbl[][])
                  }
                  frame 5 {
                    n236 = global read "_RT Global.vi" "Q2 Res Hi"() -> (w436:dbl[][])
                  }
                  frame 6 {
                    n237 = global read "_RT Global.vi" "Q1 Res Med"() -> (w437:dbl[][])
                  }
                  frame 7 {
                    n238 = global read "_RT Global.vi" "Q2 Res Med"() -> (w438:dbl[][])
                  }
                  frame 8 {
                    n239 = global read "_RT Global.vi" "Q1 Res Lo"() -> (w439:dbl[][])
                  }
                  frame 9 {
                    n240 = global read "_RT Global.vi" "Q2 Res Lo"() -> (w440:dbl[][])
                  }
                  frame 10 {
                    n241 = global read "_RT Global.vi" "Q1 -Res Hi"() -> (w441:dbl[][])
                  }
                  frame 11 {
                    n242 = global read "_RT Global.vi" "Q2 -Res Hi"() -> (w442:dbl[][])
                  }
                  frame 12 {
                    n243 = global read "_RT Global.vi" "Q1 -Res Med"() -> (w443:dbl[][])
                  }
                  frame 13 {
                    n244 = global read "_RT Global.vi" "Q2 -Res Med"() -> (w444:dbl[][])
                  }
                  frame 14 {
                    n245 = global read "_RT Global.vi" "Q1 -Res Lo"() -> (w445:dbl[][])
                  }
                  frame 15 {
                    n246 = global read "_RT Global.vi" "Q2 -Res Lo"() -> (w446:dbl[][])
                  }
                }
                n247 = Flatten To String(anything=w424) -> (data string=w427:string)  [unwired: 1 in, 4 out]
                n248 = Bundle By Name(cluster=w430, "Rt Loop Events"=RT_Loop_Events."Send Reply", "Info"=w427) -> (w429:T12)
              }
              frame "IE" {
                # "Set Igore Lost Communication Error Flag\n0 = false\n1 = true (ignore error)"
                n249 = call <vilib>:"Trim Whitespace.vi"("string"=w450) -> ("trimmed string"=w449:string)  [unwired: 1 in]
                n250 = Not Equal?(x=w449, y="0") -> (x != y?=w447:bool)
                n251 = global write "_RT Global.vi" "IgnoreError"(w447) -> ()
                n252 = Bundle By Name(cluster=w453, "Rt Loop Events"=RT_Loop_Events."Send Reply") -> (w452:T12)
              }
              frame "MM" {
                # "Set Maximum Mass"
                n253 = global read "_RT Global.vi" "Max Mass"() -> (w458:dbl)
                n254 = Unflatten From String(type=w458, binary string=w459) -> (error out=w454:errorcluster)  [unwired: 1 in, 4 out]
                n255 = Bundle By Name(cluster=w456, "Rt Loop Events"=RT_Loop_Events."Send Reply", "error"=w454) -> (w455:T12)
              }
              frame "OG" {
                # "Get Startup Options"
                n256 = global read "_RT Global.vi" "StartupOptions"() -> (w461:T18)
                n257 = Flatten To String(anything=w461) -> (data string=w460:string)  [unwired: 1 in, 4 out]
                n258 = Bundle By Name(cluster=w463, "Rt Loop Events"=RT_Loop_Events."Send Reply", "Info"=w460) -> (w462:T12)
              }
              frame "OS" {
                # "Set Startup Options"
                n259 = global read "_RT Global.vi" "StartupOptions"() -> (w473:T18)
                n260 = Unflatten From String(type=w473, binary string=w465) -> (value=w472:T18)  [unwired: 1 in, 4 out]
                n261 = global write "_RT Global.vi" "StartupOptions"(w472) -> ()
                n262 = call "_RT Open Preference File.vi"() -> ("error"=w471:errorcluster, "refnum"=w470:T17)  [unwired: 6 out]
                n263 = call-poly <vilib>:"Write Key.vi"("section"="RT", "error in (no error)"=w471, "value"=w465, "key"="SUOpt", "refnum"=w470) -> ("error out"=w466:errorcluster, "refnum out"=w467:T17)  [unwired: 1 in, 4 out]
                n264 = call <vilib>:"Close Config Data.vi"("error in (no error)"=w466, "refnum"=w467) -> ()  [unwired: 1 in, 9 out]
                n265 = Bundle By Name(cluster=w475, "Rt Loop Events"=RT_Loop_Events."Send Reply") -> (w474:T12)
              }
              frame "P1" {
                # "Set COR POL, CUR POL for Latch2"
                n266 = Type Cast(type=u16 0, x=w483) -> (*(type *) &x=w477:u16)
                n267 = call "_FPGA Set Digi Line.vi"("States"=w477, "Line (Set Latch1)"=_RW_Status."Set Latch2" ("Write Mode (Do Write)")) -> ("error out"=w478:errorcluster)  [unwired: 2 in, 3 out]
                n268 = Bundle By Name(cluster=w480, "Rt Loop Events"=RT_Loop_Events."Send Reply", "error"=w478) -> (w479:T12)
              }
              frame "P2" {
                # "Set S1 POL, S2 POL for Latch3"
                n269 = Type Cast(type=u16 0, x=w491) -> (*(type *) &x=w485:u16)
                n270 = call "_FPGA Set Digi Line.vi"("States"=w485, "Line (Set Latch1)"=_RW_Status."Set Latch3" ("Write Mode (Do Write)")) -> ("error out"=w486:errorcluster)  [unwired: 2 in, 3 out]
                n271 = Bundle By Name(cluster=w488, "Rt Loop Events"=RT_Loop_Events."Send Reply", "error"=w486) -> (w487:T12)
              }
              frame "P3" {
                # "Set CEM POL for Latch4"
                n272 = Type Cast(type=u16 0, x=w499) -> (*(type *) &x=w493:u16)
                n273 = call "_FPGA Set Digi Line.vi"("States"=w493, "Line (Set Latch1)"=_RW_Status."Set Latch4" ("Write Mode (Do Write)")) -> ("error out"=w494:errorcluster)  [unwired: 2 in, 3 out]
                n274 = Bundle By Name(cluster=w496, "Rt Loop Events"=RT_Loop_Events."Send Reply", "error"=w494) -> (w495:T12)
              }
              frame "RA" {
                # "Read ADC"
                n275 = call "_FPGA Read ADC.vi"() -> ("error out"=w503:errorcluster, "Running"=w501:bool, "ADC Values"=w502:i32[])  [unwired: 3 in, 4 out]
                n276 = local write "Running"(w501) -> ()
                n277 = Bundle By Name(cluster=w506, "Rt Loop Events"=RT_Loop_Events."Send Reply", "Data Array"=w502, "error"=w503) -> (w505:T12)
              }
              frame "RP" {
                # "Toggle Roughing Pump"
                n278 = Not Equal?(x=w508, y="0") -> (x != y?=w509:bool)
                n279 = Boolean To (0,1)(Boolean=w509) -> (0, 1=w507:i16)
                n280 = call "_FPGA Set Digi Line.vi"("States"=w507, "Line (Set Latch1)"=_RW_Status."RP ON" ("Write Mode (Do Write)")) -> ("error out"=w511:errorcluster)  [unwired: 2 in, 3 out]
                n281 = Bundle By Name(cluster=w513, "Rt Loop Events"=RT_Loop_Events."Send Reply", "error"=w511) -> (w512:T12)
              }
              frame "RS" {
                w529 = u8 0 ("default (0 I32)")
                # "Toggle the startup/shut down"
                n282 = call <vilib>:"Trim Whitespace.vi"("string"=w532) -> ("trimmed string"=w531:string)  [unwired: 1 in]
                n283 = global read "_RT Global.vi" "InstrState"() -> (w518:T2)
                n284 = Decimal String To Number(string=w531, default (0L)=w529) -> (number=w530:u8)  [unwired: 2 out]
                n285 = In Range and Coerce(upper limit=u8 2, x=w530, lower limit=w529) -> (coerced(x)=w522:u8)  [unwired: 1 out]
                n286 = Not Equal?(x=w518, y=_RT_Instrument_State."Starting Up") -> (x != y?=w524:bool)
                n287 = Not Equal?(x=w518, y=_RT_Instrument_State."Turbo Startup") -> (x != y?=w519:bool)
                n288 = Not Equal?(x=w518, y=_RT_Instrument_State."Shutting Down") -> (x != y?=w516:bool)
                n289 = Not Equal?(x=w522, y=u8 1) -> (x != y?=w523:bool)
                n290 = Compound Arithmetic op=AND(w524, w519, w516) -> (w520:bool)
                n291 = Or(x=w523, y=w520) -> (x .or. y?=w521:bool)
                n292 = case shown="True" w521 {
                  tunnel: w522 -> [_ w537]
                  frame False {
                  }
                  frame True {
                    n293 = Greater Than 0?(x=w537) -> (x > 0?=w536:bool)
                    n294 = global write "_RT Global.vi" "StartupMode"(w537) -> ()
                    n295 = case shown="True" w536 {
                      frame False {
                      }
                      frame True {
                        n296 = call "_FPGA Turn LC Pump Off.vi"() -> ()  [unwired: 2 in]
                      }
                    }
                  }
                }
                n297 = Bundle By Name(cluster=w535, "Rt Loop Events"=RT_Loop_Events."Send Reply") -> (w534:T12)
              }
              frame "RU" {
                w539 = T4[] []  # Parameters
                # "Do a Run-Time Update"
                n298 = xnode "Read/Write Control"("FPGA VI Reference In"=w543) -> ("error out"=w542:errorcluster, "Running"=w538:bool)  [unwired: 1 in, 1 out]
                n299 = Unflatten From String(type=w539, binary string=w547) -> (value=w541:T4[])  [unwired: 1 in, 4 out]
                n300 = local write "Running"(w538) -> ()
                n301 = case shown="True" w538 {
                  tunnel: w542 -> [w548 w551]
                  tunnel: w541 -> [_ w549]
                  tunnel: [w548 w550] -> w540
                  frame False {
                  }
                  frame True {
                    n302 = call "_FPGA Runtime Update.vi"("error in"=w551, "Parameters"=w549) -> ("error out"=w550:errorcluster)  [unwired: 1 in, 4 out]
                  }
                }
                n303 = Bundle By Name(cluster=w545, "Rt Loop Events"=RT_Loop_Events."Send Reply", "error"=w540) -> (w544:T12)
              }
              frame "RV" {
                # "Read VAC Gauge"
                n304 = call "_FPGA Read Data.vi"("Read Mode (Do Read)"=_RW_Status."Read VAC" ("R/W Status")) -> ("error out"=w552:errorcluster, "Data"=w553:u32)  [unwired: 4 in, 1 out]
                n305 = Build Array(w553) -> (w555:u32[])
                n306 = Bundle By Name(cluster=w557, "Rt Loop Events"=RT_Loop_Events."Send Reply", "Data Array"=w555, "error"=w552) -> (w556:T12)
              }
              frame "SC" {
                # "Set Configuration"
                n307 = global read "_RT Global.vi" "Configuration 2"() -> (w578:T10)
                n308 = Unflatten From String(type=w578, binary string=w579) -> (value=w564:T10, error out=w567:errorcluster)  [unwired: 1 in, 3 out]
                n309 = Unbundle By Name(w564) -> ("Instrument"=w566:string[])
                n310 = Current VI's Path() -> (path=w572:path)
                n311 = Strip Path(path=w572) -> (stripped path=w573:path)  [unwired: 1 out]
                n312 = Strip Path(path=w573) -> (stripped path=w574:path)  [unwired: 1 out]
                n313 = Index Array(array=w566, index=2) -> (element=w560:string)
                n314 = Build Path(base path=w574, name or relative path="Config" ("key")) -> (appended path=w570:path)
                n315 = Match Pattern(string=w560, regular expression="Simulation") -> (offset past match=w563:i32)  [unwired: 4 out]
                n316 = call "_Convert Model Name.vi"("Model"=w560) -> ("SingleSource"=w559:bool)  [unwired: 1 in, 1 out]
                n317 = global write "_RT Global.vi" "Configuration 2"(w564) -> ()
                n318 = Greater Or Equal To 0?(x=w563) -> (x >= 0?=w561:bool)
                n319 = Write to Binary File(file (use dialog)=w570, data=w564, error in=w567) -> (refnum out=w568:refnum<file>, error out=w569:errorcluster)  [unwired: 4 out]
                n320 = global write "_RT Global.vi" "Single Source"(w559) -> ()
                n321 = global write "_RT Global.vi" "Simulation"(w561) -> ()
                n322 = Close File(refnum=w568, error in=w569) -> ()  [unwired: 2 out]
                n323 = Bundle By Name(cluster=w576, "Rt Loop Events"=RT_Loop_Events."Send Reply") -> (w575:T12)
              }
              frame "SL" {
                # "Set LC Outputs"
                n324 = Type Cast(type=u16 0, x=w582) -> (*(type *) &x=w581:u16)
                n325 = call "_FPGA Write Data.vi"("Write Mode (Do Write)"=_RW_Status."Set LC Out", "Address"=w581) -> ("error out"=w580:errorcluster)  [unwired: 4 in, 2 out]
                n326 = Bundle By Name(cluster=w586, "Rt Loop Events"=RT_Loop_Events."Send Reply", "error"=w580) -> (w585:T12)
              }
              frame "SO" {
                # "Set Oscillator"
                n327 = Unflatten From String(type=u32[] [], binary string=w592) -> (value=w595:u32[])  [unwired: 1 in, 4 out]
                n328 = xnode "Read/Write Control"("FPGA VI Reference In"=w597) -> ("error out"=w596:errorcluster, "Running"=w591:bool)  [unwired: 1 in, 1 out]
                n329 = local write "Running"(w591) -> ()
                n330 = Index Array(array=w595) -> (element #1=w590:u32, element #2=w589:u32, element #3=w588:u32)  [unwired: 3 in]
                n331 = call "_FPGA Set Oscillator.vi"("Param 3"=w588, "error in"=w596, "Param 2"=w589, "Param 1"=w590) -> ("error out"=w594:errorcluster)  [unwired: 1 in, 3 out]
                n332 = Bundle By Name(cluster=w599, "Rt Loop Events"=RT_Loop_Events."Send Reply", "error"=w594) -> (w598:T12)
              }
              frame "SP" {
                # "Set PIC"
                n333 = Unflatten From String(type=u32[] [], binary string=w612) -> (value=w606:u32[])  [unwired: 1 in, 4 out]
                n334 = xnode "Read/Write Control"("FPGA VI Reference In"=w608) -> ("error out"=w607:errorcluster, "Running"=w604:bool)  [unwired: 1 in, 1 out]
                n335 = local write "Running"(w604) -> ()
                n336 = case shown="False" w604 {
                  tunnel: w607 -> [w618 w620]
                  tunnel: w606 -> [w616 _]
                  tunnel: [w617 w619] -> w603
                  tunnel: [w613 _] -> w602
                  frame False {
                    n337 = Index Array(array=w616) -> (element #1=w615:u32, element #2=w614:u32)  [unwired: 2 in]
                    n338 = call "_FPGA Set PIC.vi"("error in"=w618, "Param 2"=w614, "Param 1"=w615) -> ("error out"=w617:errorcluster, "Data"=w613:u32)  [unwired: 2 in, 1 out]
                  }
                  frame True {
                    n339 = call "_Construct Error Cluster.vi"("error in"=w620, "reason"="Cannot send command to PIC because the instrument is busy.") -> ("error out"=w619:errorcluster)  [unwired: 2 in, 3 out]
                  }
                }
                n340 = Build Array(w602) -> (w601:u32[])
                n341 = Bundle By Name(cluster=w610, "Rt Loop Events"=RT_Loop_Events."Send Reply", "Data Array"=w601, "error"=w603) -> (w609:T12)
              }
              frame "SS" {
                # "Send Serial Command"
                n342 = Unflatten From String(type=T15 {"Port Type"=0, "baud rate (9600)"=9600, "data bits (8)"=8, "stop bits (1)"=10, "parity (0:none)"=0, "DoRead"=FALSE, "Command"=""} ("Serial Command"), binary string=w632) -> (value=w626:T15)  [unwired: 1 in, 4 out]
                n343 = xnode "Read/Write Control"("FPGA VI Reference In"=w628) -> ("error out"=w627:errorcluster, "Running"=w625:bool)  [unwired: 1 in, 1 out]
                n344 = local write "Running"(w625) -> ()
                n345 = case shown="False" w625 {
                  tunnel: w627 -> [w635 w638]
                  tunnel: w626 -> [w634 _]
                  tunnel: [w636 w637] -> w624
                  tunnel: [w633 _] -> w622
                  frame False {
                    n346 = call "_FPGA Send Serial.vi"("error in"=w635, "Serial Command"=w634) -> ("error out"=w636:errorcluster, "Reply"=w633:string)  [unwired: 2 in, 2 out]
                  }
                  frame True {
                    n347 = call "_Construct Error Cluster.vi"("error in"=w638, "reason"="Cannot send command to serial port because the instrument is busy.") -> ("error out"=w637:errorcluster)  [unwired: 2 in, 3 out]
                  }
                }
                n348 = Bundle By Name(cluster=w630, "Rt Loop Events"=RT_Loop_Events."Send Reply", "Info"=w622, "error"=w624) -> (w629:T12)
              }
              frame "ST" {
                # "Start a Run"
                n349 = global read "_RT Global.vi" "FPGA semaphore"() -> (w642:T9)
                n350 = Unbundle By Name(w645) -> ("Parameter"=w647:T3)
                n351 = Unflatten From String(type=w647, binary string=w648) -> (value=w640:T3)  [unwired: 1 in, 4 out]
                n352 = stacked-sequence {
                  tunnel: w641 -> [_ w656 _ _]
                  tunnel: w640 -> [_ w657 _ _]
                  tunnel: [_ w662 _ _] -> w643
                  tunnel: w642 -> [w655 _ _ w679]
                  frame #0 {
                    n353 = call <vilib>:"Acquire Semaphore.vi"("ms timeout (-1)"=2000, "semaphore"=w655) -> ("timed out"=w649:bool)  [unwired: 1 in, 4 out]
                    n354 = local read "Running"() -> (w652:bool)
                    n355 = global read "_RT Global.vi" "InstrState"() -> (w653:T2)
                    n356 = Format Into String(format string="Start Run: Instr State = %s; FPGA Running = %s;  Time Out = %s.", w653, w652, w649) -> (resulting string=w650:string)  [unwired: 2 in, 1 out]
                    n357 = call "_RT Event.vi"("Event"=w650) -> ()  [unwired: 2 in, 5 out]
                  }
                  frame #1 {
                    n358 = call "_Update Parameter Data.vi"("Parameter"=w657) -> ("error out"=w658:errorcluster, "RF Only"=w659:bool)  [unwired: 2 in, 3 out]
                    n359 = local read "Ready"() -> (w660:bool)
                    n360 = Or(x=w659, y=w660) -> (x .or. y?=w661:bool)
                    n361 = case shown="True" w661 {
                      tunnel: w656 -> [_ w670]
                      tunnel: w657 -> [_ w672]
                      tunnel: [w664 w669] -> w662
                      tunnel: w658 -> [_ w666]
                      frame False {
                        n362 = call "_Construct Error Cluster.vi"("reason"="8016: A run is in progress or system is not ready.", "errorCode"=8016) -> ("error out"=w664:errorcluster)  [unwired: 2 in, 3 out]
                      }
                      frame True {
                        n363 = Unbundle By Name(w672) -> ("RunMode"=w667:i32)
                        "RunMode" <- w667
                        n364 = case shown="3, 6, 7" w667 {
                          tunnel: w666 -> [w673 w674]
                          tunnel: [w673 w674] -> w671
                          frame 0, Default {
                          }
                          frame 3, 6, 7 {
                            n365 = call "_FPGA Read Counter.vi"() -> ()  [unwired: 2 in, 4 out]
                          }
                        }
                        n366 = case shown="No Error" w671 {
                          selector: w671 -> [_ w677]
                          tunnel: w670 -> [w676 _]
                          tunnel: [_ w677] -> w669
                          tunnel: [w675 _] -> w668
                          frame No Error {
                            w675 = TRUE ("Start")
                            n367 = xnode "Read/Write Control"("FPGA VI Reference In"=w676, "Start"=w675) -> ()  [unwired: 1 in, 2 out]
                          }
                          frame Error {
                          }
                        }
                        "Running" <- w668
                      }
                    }
                  }
                  frame #2 {
                    n368 = Wait (ms)(milliseconds to wait=u32 180) -> ()  [unwired: 1 out]
                  }
                  frame #3 {
                    n369 = call <vilib>:"Release Semaphore.vi"("semaphore"=w679) -> ()  [unwired: 1 in, 6 out]
                  }
                }
                n370 = Bundle By Name(cluster=w645, "Rt Loop Events"=RT_Loop_Events."Send Reply", "Parameter"=w640, "error"=w643) -> (w644:T12)
              }
              frame "TT" {
                w690 = u16 405 ("Address")
                # "Run Table Test"
                n371 = Unflatten From String(type=u32[] [], binary string=w695) -> (value=w693:u32[])  [unwired: 1 in, 4 out]
                n372 = Index Array(array=w693) -> (element #1=w692:u32, element #2=w689:u32)  [unwired: 2 in]
                n373 = Increment(x=w690) -> (x+1=w687:u16)
                n374 = call "_FPGA Write Data.vi"("Data"=w692, "Address"=w690) -> ("error out"=w691:errorcluster)  [unwired: 4 in, 2 out]
                n375 = call "_FPGA Write Data.vi"("error in"=w691, "Data"=w689, "Address"=w687) -> ("error out"=w688:errorcluster)  [unwired: 3 in, 2 out]
                n376 = xnode "Read/Write Control"("FPGA VI Reference In"=w694, "error in"=w688, "R/W Status"=_RW_Status."Table Test") -> ("FPGA VI Reference Out"=w699:refnum<k20>, "error out"=w698:errorcluster)
                n377 = xnode "Read/Write Control"("FPGA VI Reference In"=w699, "error in"=w698, "Read/Write"=TRUE ("Data Written")) -> ("error out"=w700:errorcluster)  [unwired: 1 out]
                n378 = call "_FPGA Wait Done.vi"("error in"=w700, "Indicator"=_FPGA_Indicator."Done") -> ("error out"=w686:errorcluster)  [unwired: 3 in, 2 out]
                n379 = Increment(x=w687) -> (x+1=w683:u16)
                n380 = call "_FPGA Read Data.vi"("error in"=w686, "Address"=w683) -> ("error out"=w685:errorcluster, "Data"=w681:u32)  [unwired: 3 in, 1 out]
                n381 = Increment(x=w683) -> (x+1=w684:u16)
                n382 = call "_FPGA Read Data.vi"("error in"=w685, "Address"=w684) -> ("error out"=w682:errorcluster, "Data"=w680:u32)  [unwired: 3 in, 1 out]
                n383 = Build Array(w681, w680) -> (w697:u32[])
                n384 = Bundle By Name(cluster=w705, "Rt Loop Events"=RT_Loop_Events."Send Reply", "Data Array"=w697, "error"=w682) -> (w704:T12)
              }
              frame "UT" {
                # "Update a Calibration/Resolution Table"
                n385 = Unflatten From String(type=cluster{"Type":u16, "Table":dbl[][]} {"Type"=0, "Table"=[]} ("Calibration"), binary string=w709) -> (value=w710:cluster{"Type":u16, "Table":dbl[][]})  [unwired: 1 in, 4 out]
                n386 = Unbundle By Name(w710) -> ("Type"=w708:u16, "Table"=w707:dbl[][])
                n387 = stacked-sequence {
                  tunnel: [_ w752] -> w713
                  tunnel: w708 -> [w718 w751]
                  tunnel: w707 -> [w716 _]
                  frame #0 {
                    n388 = case shown="0, Default" w718 {
                      tunnel: ["Cal" ("key") "Cal2" ("key") "Cal3" ("key") "Cal4" ("key") "Res" ("key") "Res2" ("key") "Res3" ("key") "Res4" ("key") "Res5" ("key") "Res6" ("key") "Res7" ("key") "Res8" ("key") "Res9" ("key") "Res10" ("key") "Res11" ("key") "Res12" ("key")] -> w717
                      frame 0, Default {
                      }
                      frame 1 {
                      }
                      frame 2 {
                      }
                      frame 3 {
                      }
                      frame 4 {
                      }
                      frame 5 {
                      }
                      frame 6 {
                      }
                      frame 7 {
                      }
                      frame 8 {
                      }
                      frame 9 {
                      }
                      frame 10 {
                      }
                      frame 11 {
                      }
                      frame 12 {
                      }
                      frame 13 {
                      }
                      frame 14 {
                      }
                      frame 15 {
                      }
                    }
                    n389 = case shown="3" w718 {
                      tunnel: w716 -> [w719 w720 w721 w722 w723 w724 w725 w726 w727 w728 w729 w730 w731 w732 w733 w734]
                      frame 0, Default {
                        n390 = global write "_RT Global.vi" "Q1 Cal"(w719) -> ()
                      }
                      frame 1 {
                        n391 = global write "_RT Global.vi" "Q2 Cal"(w720) -> ()
                      }
                      frame 2 {
                        n392 = global write "_RT Global.vi" "Q1 -Cal"(w721) -> ()
                      }
                      frame 3 {
                        n393 = global write "_RT Global.vi" "Q2 -Cal"(w722) -> ()
                      }
                      frame 4 {
                        n394 = global write "_RT Global.vi" "Q1 Res Hi"(w723) -> ()
                      }
                      frame 5 {
                        n395 = global write "_RT Global.vi" "Q2 Res Hi"(w724) -> ()
                      }
                      frame 6 {
                        n396 = global write "_RT Global.vi" "Q1 Res Med"(w725) -> ()
                      }
                      frame 7 {
                        n397 = global write "_RT Global.vi" "Q2 Res Med"(w726) -> ()
                      }
                      frame 8 {
                        n398 = global write "_RT Global.vi" "Q1 Res Lo"(w727) -> ()
                      }
                      frame 9 {
                        n399 = global write "_RT Global.vi" "Q2 Res Lo"(w728) -> ()
                      }
                      frame 10 {
                        n400 = global write "_RT Global.vi" "Q1 -Res Hi"(w729) -> ()
                      }
                      frame 11 {
                        n401 = global write "_RT Global.vi" "Q2 -Res Hi"(w730) -> ()
                      }
                      frame 12 {
                        n402 = global write "_RT Global.vi" "Q1 -Res Med"(w731) -> ()
                      }
                      frame 13 {
                        n403 = global write "_RT Global.vi" "Q2 -Res Med"(w732) -> ()
                      }
                      frame 14 {
                        n404 = global write "_RT Global.vi" "Q1 -Res Lo"(w733) -> ()
                      }
                      frame 15 {
                        n405 = global write "_RT Global.vi" "Q2 -Res Lo"(w734) -> ()
                      }
                    }
                    n406 = call "_Save RT Table.vi"("Table"=w716, "key"=w717) -> ()  [unwired: 1 in, 5 out]
                  }
                  frame #1 {
                    n407 = call "_Update Cal or Res Data.vi"("Table Type"=w751) -> ("error out"=w752:errorcluster)  [unwired: 2 in, 4 out]
                  }
                }
                n408 = Bundle By Name(cluster=w715, "Rt Loop Events"=RT_Loop_Events."Send Reply", "error"=w713) -> (w712:T12)
              }
              frame Default {
                n409 = Format Into String(format string="Message Type: %s, not recognized by firmware command receiver.", w759) -> (resulting string=w757:string)  [unwired: 2 in, 1 out]
                n410 = call "_Construct Error Cluster.vi"("reason"=w757) -> ("error out"=w753:errorcluster)  [unwired: 3 in, 3 out]
                n411 = Bundle By Name(cluster=w755, "Rt Loop Events"=RT_Loop_Events."Send Reply", "error"=w753) -> (w754:T12)
              }
            }
            n412 = local write "Disconnection#"(u8 0 ("Disconnection#")) -> ()
          }
          frame True {
            # "No command received from the host at this time,\nor the host has been disconnected."
            n413 = local read "Disconnection#"() -> (w764:u8)
            n414 = Greater?(x=w764, y=u8 2) -> (0:w761:bool)
            n415 = Wait Until Next ms Multiple(millisecond multiple=u32 380 ("milliseconds to wait")) -> ()  [unwired: 1 out]
            n416 = case shown="True" w761 {
              tunnel: w764 -> [w770 _]
              tunnel: w763 -> [_ w773]
              tunnel: [RT_Loop_Events."Wait for Command" ("Rt Loop Events") RT_Loop_Events."Wait for Connection" ("Rt Loop Events")] -> w762
              frame False {
                n417 = Increment(x=w770) -> (x+1=→"Disconnection#":u8)
              }
              frame True {
                n418 = TCP Close Connection(connection ID=w773, abort (F)=TRUE) -> ()  [unwired: 1 in, 2 out]
                "Connected?" <- FALSE ("Connected?")
              }
            }
            n419 = Bundle By Name(cluster=w767, "Rt Loop Events"=w762) -> (w766:T12)
          }
        }
      }
      frame "Send Reply" {
        w779 = i32[] []  # Data Array
        w777 = errorcluster {"status"=FALSE, "code"=0, "source"=""}  # error
        w780 = ""  # Info
        # "Send a reply back to the host after receiving each command"
        n420 = Unbundle By Name(w782) -> ("Connection ID"=w784:refnum<k5>, "Info"=w785:string, "Data Array"=w788:i32[], "error"=w778:errorcluster)
        n421 = Bundle("Info"=w785, "Data Array"=w788, "error"=w778) -> (w776:T19)  [unwired: 1 out]
        n422 = Flatten To String(anything=w776) -> (data string=w786:string)  [unwired: 1 in, 4 out]
        n423 = call "_TCP Msg Write.vi"("Data Stream"=w786, "Message Type"="RE" ("Name"), "connection ID"=w784) -> ()  [unwired: 2 in, 7 out]
        n424 = Bundle By Name(cluster=w782, "Rt Loop Events"=RT_Loop_Events."Wait for Command", "Info"=w780, "Data Array"=w779, "error"=w777) -> (w781:T12)
      }
    }
  }
  n425 = Greater Or Equal To 0?(x=w9) -> (x >= 0?=w7:bool)
  n426 = Greater Than 0?(x=w19) -> (x > 0?=w18:bool)
  n427 = case shown="False" w18 {
    tunnel: [_RT_Instrument_State."Initializing" ("InstrState") _RT_Instrument_State."Starting Up" ("InstrState")] -> w33
    frame False {
    }
    frame True {
      n428 = global write "_RT Global.vi" "StartupMode"(u8 0 ("StartupMode")) -> ()
    }
  }
  n429 = call "_Convert Model Name.vi"("Model"=w6) -> ("SingleSource"=w5:bool)  [unwired: 1 in, 1 out]
  n430 = global write "_RT Global.vi" "Simulation"(w7) -> ()
  n431 = global write "_RT Global.vi" "Single Source"(w5) -> ()
  n432 = while {
    tunnel: w4 -> [w792]
    shift-right: [w796] -> _
    shift-left: w33 -> [w795]
    i -> [w794]
    stop <- FALSE stop-if-true
    n433 = case shown="\"Going to Standby\"" w795 {
      selector: w795 -> [_ w815 _ _ w837 _ _ _ w865 _ w890 w907 _ _ w998 w1025 w1044 w1077 _ _]
      tunnel: w792 -> [_ _ _ _ _ _ _ _ _ _ _ _ w926 _ _ _ _ _ _ _]
      tunnel: [_RT_Instrument_State."Mass Spectrometer is Off" ("InstrState") w814 w819 _RT_Instrument_State."Roughing Pump Ready" ("InstrState") w838 w849 _RT_Instrument_State."Initializing" ("t") _RT_Instrument_State."Going to Standby" ("t") w864 _RT_Instrument_State."24V Standby" ("InstrState") w889 w906 w927 _RT_Instrument_State."Ready" ("InstrState") w1000 w1026 w1047 w1074 w1088 _RT_Instrument_State."Shutting Down" ("t")] -> w796
      tunnel: w794 -> [_ _ _ _ _ _ _ _ _ _ _ _ _ _ w993 _ w1042 _ _ _]
      frame "Initializing" {
        w800 = T22 11 items=["Same", "Empty", "VacFail", "Cancel", "CheckGas", "EleFail", "Probe1Fail", "Probe2Fail", "HeaterFail", "DoorOpen", "CheckComm", "PressStart"] ("Line2Msg (same)")
        w801 = T23 2 items=["Same", "Empty", "Connected", "Starting", "Stopping", "Action", "On", "Service", "Call", "Acquiring", "Source"] ("Line1Msg (same)")
        w803 = FALSE ("Connected?")
        # "Going to System Off State"
        n434 = call "_FPGA Set LEDs.vi"("LED Command"=_LED_States."Off BRP") -> ("error out"=w805:errorcluster)  [unwired: 3 in, 3 out]
        n435 = Wait (ms)(milliseconds to wait=u32 1800) -> ()  [unwired: 1 out]
        n436 = call "_FPGA Set LCD Msg.vi"("error in"=w805, "Line2Msg (same)"=w800, "Line1Msg (same)"=w801) -> ("error out"=w798:errorcluster)  [unwired: 4 in, 2 out]
        n437 = call "_FPGA Send LCD.vi"("error in (no error)"=w798, "Command"=_RT_LED_Num."ReadKey" ("LED#")) -> ()  [unwired: 2 in, 5 out]
        n438 = global write "_RT Global.vi" "StartupMode"(u8 2 ("StartupMode")) -> ()
        n439 = local write "Running"(FALSE ("Connected?")) -> ()
        n440 = call "_RT Event.vi"("Event"="Mass Spectrometer is OFF. Power Connected") -> ()  [unwired: 2 in, 5 out]
        "Ready" <- w803
        "Fault" <- w803
      }
      frame "Mass Spectrometer is Off" {
        # "Wait for the start up command"
        n441 = call "_FPGA Read Key.vi"("CurStartupMode (0)"=u8 2, "ForStart (F)"=TRUE) -> ("Key Pressed"=w812:bool)  [unwired: 3 in, 3 out]
        n442 = Select(t=_RT_Instrument_State."Starting Up", s=w812, f=w815) -> (s? t:f=w814:T2)
      }
      frame "Starting Up" {
        w817 = FALSE ("Status LED")
        # "Start a startup sequence"
        n443 = call "_FPGA Send LCD.vi"("Command"=_RT_LED_Num."ReadKey" ("LED#")) -> ("error out"=w816:errorcluster)  [unwired: 4 in, 3 out]
        n444 = call "_Update Start Up.vi"("error in (no error)"=w816) -> ("Next InstrState"=w819:T2)  [unwired: 2 in, 4 out]
        n445 = local write "Ready"(w817) -> ()
        n446 = local write "Fault"(w817) -> ()
      }
      frame "Going to Standby" {
        w823 = T23 8 items=["Same", "Empty", "Connected", "Starting", "Stopping", "Action", "On", "Service", "Call", "Acquiring", "Source"] ("Line1Msg (same)")
        n447 = call "_FPGA Read ADC.vi"() -> ("error out"=w820:errorcluster)  [unwired: 3 in, 6 out]
        n448 = call "_FPGA Check Source ID.vi"("error in (no error)"=w820) -> ("Source ID OK"=w825:bool)
        n449 = call "_FPGA Set Parameters.vi"("ExhaustGas (on)"=FALSE, "error in"=w820, "HSID Temp (on)"=w825) -> ("error out"=w827:errorcluster)  [unwired: 6 in, 2 out]
        n450 = call "_FPGA Set LEDs.vi"("error in (no error)"=w827, "LED Command"=_LED_States."Off BRP") -> ("error out"=w826:errorcluster)  [unwired: 2 in, 3 out]
        n451 = call "_FPGA Set LEDs.vi"("error in (no error)"=w826, "LED Command"=_LED_States."Solid P") -> ("error out"=w831:errorcluster)  [unwired: 2 in, 3 out]
        n452 = call "_FPGA Set LCD Msg.vi"("error in"=w831, "Line1Msg (same)"=w823) -> ("error out"=w832:errorcluster)  [unwired: 5 in, 2 out]
        n453 = call "_RT Event.vi"("Event"="Roughing Pump Ready state.") -> ()  [unwired: 2 in, 5 out]
        n454 = call "_FPGA Send LCD.vi"("error in (no error)"=w832, "Command"=_RT_LED_Num."ReadKey" ("LED#")) -> ()  [unwired: 3 in, 4 out]
        n455 = global write "_RT Global.vi" "StartupMode"(u8 1 ("StartupMode")) -> ()
        n456 = local write "Ready"(FALSE ("Status LED")) -> ()
        n457 = local write "Fault"(TRUE ("Fault")) -> ()
      }
      frame "Roughing Pump Ready" {
        n458 = global read "_RT Global.vi" "StartupMode"() -> (w836:u8)
        n459 = case shown="1, Default" w836 {
          tunnel: [_RT_Instrument_State."Turbo Startup" ("InstrState") w842 _RT_Instrument_State."Shutting Down" ("InstrState")] -> w838
          tunnel: w837 -> [_ w840 _]
          frame 0 {
            # "Continue the startup sequence"
          }
          frame 1, Default {
            # "Wait for Start key to restart the system"
            n460 = call "_FPGA Read Key.vi"("CurStartupMode (0)"=u8 1, "ForStart (F)"=TRUE) -> ("Key Pressed"=w845:bool)  [unwired: 3 in, 3 out]
            n461 = Select(t=_RT_Instrument_State."Turbo Startup", s=w845, f=w840) -> (s? t:f=w842:T2)
          }
          frame 2 {
            # "Received a shutdown command"
          }
        }
      }
      frame "Turbo Startup" {
        # "Continue the startup sequence"
        n462 = call "_FPGA Send LCD.vi"("Command"=_RT_LED_Num."ReadKey" ("LED#")) -> ("error out"=w847:errorcluster)  [unwired: 4 in, 3 out]
        n463 = call "_Update Start Up Turbo.vi"("error in (no error)"=w847) -> ("Next InstrState"=w849:T2)  [unwired: 2 in, 4 out]
      }
      frame "Turning Power Off" {
        w850 = T23 4 items=["Same", "Empty", "Connected", "Starting", "Stopping", "Action", "On", "Service", "Call", "Acquiring", "Source"] ("Line1Msg (same)")
        n464 = call "_FPGA Set LCD Msg.vi"("Line1Msg (same)"=w850) -> ()  [unwired: 6 in, 3 out]
        n465 = local write "Ready"(FALSE ("Status LED")) -> ()
        n466 = local write "Fault"(TRUE ("Status LED")) -> ()
        n467 = Wait (ms)(milliseconds to wait=u32 1800) -> ()  [unwired: 1 out]
      }
      frame "Turning Turbo Off" {
        n468 = stacked-sequence {
          frame #0 {
            n469 = Wait (ms)(milliseconds to wait=u32 1800) -> ()  [unwired: 1 out]
          }
          frame #1 {
            n470 = call "_FPGA Send LCD.vi"("Command"=_RT_LED_Num."ReadKey" ("LED#")) -> ()  [unwired: 4 in, 4 out]
          }
        }
        n471 = local write "Ready"(FALSE ("Status LED")) -> ()
        n472 = local write "Fault"(TRUE ("Status LED")) -> ()
      }
      frame "Turbopump Ready" {
        w861 = T23 5 items=["Same", "Empty", "Connected", "Starting", "Stopping", "Action", "On", "Service", "Call", "Acquiring", "Source"] ("Line1Msg (same)")
        n473 = global read "_RT Global.vi" "StartupMode"() -> (w866:u8)
        n474 = local write "Fault"(TRUE ("Status LED")) -> ()
        n475 = call "_FPGA Set LCD Msg.vi"("Line1Msg (same)"=w861) -> ("error out"=w860:errorcluster)  [unwired: 6 in, 2 out]
        n476 = case shown="Default" w866 {
          tunnel: [w873 _RT_Instrument_State."Shutting Down" ("InstrState") _RT_Instrument_State."Checking Vacuum" ("InstrState")] -> w864
          tunnel: w865 -> [w870 _ _]
          tunnel: w860 -> [_ _ _]
          frame Default {
            # "Allow system to shut down from this state"
            n477 = local read "Connected?"() -> (w872:bool)
            n478 = call "_FPGA Read Key.vi"("CurStartupMode (0)"=u8 1) -> ("error out"=w867:errorcluster, "Key Pressed"=w875:bool)  [unwired: 4 in, 2 out]
            n479 = call "_FPGA System Polling.vi"("error in (no error)"=w867, "Connected?"=w872, "CurInstrState"=w870) -> ("Running"=w871:bool, "Next InstrState"=w869:T2)  [unwired: 2 in, 2 out]
            n480 = local write "Running"(w871) -> ()
            n481 = Select(t=_RT_Instrument_State."Shutting Down", s=w875, f=w869) -> (s? t:f=w873:T2)
          }
          frame 2 {
            # "Received a shutdown command"
          }
          frame 0 {
            # "Received a startup command"
          }
        }
        n482 = local write "Ready"(FALSE ("Status LED")) -> ()
      }
      frame "Go to 24V Standby" {
        w881 = T23 7 items=["Same", "Empty", "Connected", "Starting", "Stopping", "Action", "On", "Service", "Call", "Acquiring", "Source"] ("Line1Msg (same)")
        n483 = local write "Fault"(TRUE ("Status LED")) -> ()
        n484 = call "_FPGA Set LCD Msg.vi"("Line1Msg (same)"=w881) -> ("error out"=w878:errorcluster)  [unwired: 6 in, 2 out]
        n485 = global read "_RT Global.vi" "Ele On"() -> (w880:bool)
        n486 = local write "Ready"(FALSE ("Status LED")) -> ()
        n487 = case shown="True" w880 {
          tunnel: w878 -> [_ _]
          frame False {
          }
          frame True {
            # "Turn off electronics"
            n488 = call "_FPGA Toggle Electronics.vi"() -> ()  [unwired: 3 in, 6 out]
          }
        }
        n489 = call "_RT Event.vi"("Event"="Going to 24V Standby state.") -> ()  [unwired: 2 in, 5 out]
      }
      frame "Turbopump Ready-Waiting" {
        w886 = T23 8 items=["Same", "Empty", "Connected", "Starting", "Stopping", "Action", "On", "Service", "Call", "Acquiring", "Source"] ("Line1Msg (same)")
        n490 = global read "_RT Global.vi" "StartupMode"() -> (w891:u8)
        n491 = local write "Fault"(TRUE ("Status LED")) -> ()
        n492 = call "_FPGA Set LCD Msg.vi"("Line1Msg (same)"=w886) -> ("error out"=w885:errorcluster)  [unwired: 6 in, 2 out]
        n493 = case shown="Default" w891 {
          tunnel: [w896 _RT_Instrument_State."Shutting Down" ("InstrState") _RT_Instrument_State."Checking Vacuum" ("InstrState")] -> w889
          tunnel: w890 -> [w899 _ _]
          tunnel: w885 -> [_ _ _]
          frame Default {
            # "Allow system to proceed to ready from this state"
            n494 = local read "Connected?"() -> (w901:bool)
            n495 = call "_FPGA Read Key.vi"("CurStartupMode (0)"=u8 1, "ForStart (F)"=TRUE) -> ("error out"=w892:errorcluster, "Key Pressed"=w895:bool)  [unwired: 3 in, 2 out]
            n496 = call "_FPGA System Polling.vi"("error in (no error)"=w892, "Waiting (F)"=TRUE, "Connected?"=w901, "CurInstrState"=w899) -> ("Running"=w900:bool, "Next InstrState"=w894:T2)  [unwired: 1 in, 2 out]
            n497 = case shown="True" w895 {
              tunnel: [w902 _RT_Instrument_State."Checking Vacuum" ("t")] -> w896
              tunnel: w894 -> [w902 _]
              frame False {
              }
              frame True {
              }
            }
            n498 = local write "Running"(w900) -> ()
          }
          frame 2 {
            # "Received a shutdown command"
          }
          frame 0 {
            # "Received a startup command"
          }
        }
        n499 = local write "Ready"(FALSE ("Status LED")) -> ()
      }
      frame "24V Standby" {
        n500 = global read "_RT Global.vi" "StartupMode"() -> (w908:u8)
        n501 = case shown="Default" w908 {
          tunnel: [w916 _RT_Instrument_State."Shutting Down" ("InstrState") _RT_Instrument_State."Starting Up" ("InstrState")] -> w906
          tunnel: w907 -> [w914 _ _]
          frame Default {
            # "Allow system to restart from this state"
            n502 = local read "Connected?"() -> (w920:bool)
            n503 = call "_FPGA Read Key.vi"("CurStartupMode (0)"=u8 1, "ForStart (F)"=TRUE) -> ("error out"=w909:errorcluster, "Key Pressed"=w912:bool)  [unwired: 3 in, 2 out]
            n504 = call "_FPGA System Polling.vi"("error in (no error)"=w909, "Waiting (F)"=TRUE, "Connected?"=w920, "CurInstrState"=w914) -> ("Running"=w919:bool, "Next InstrState"=w915:T2)  [unwired: 1 in, 2 out]
            n505 = Not Equal?(x=w914, y=w915) -> (x != y?=w913:bool)
            n506 = Or(x=w912, y=w913) -> (x .or. y?=w911:bool)
            n507 = case shown="False" w911 {
              tunnel: [w921 _RT_Instrument_State."Starting Up" ("t")] -> w916
              tunnel: w915 -> [w921 _]
              frame False {
              }
              frame True {
                n508 = global write "_RT Global.vi" "StartupMode"(u8 0 ("StartupMode")) -> ()
              }
            }
            n509 = local write "Running"(w919) -> ()
          }
          frame 2 {
            # "Received a shutdown command"
          }
          frame 0 {
            # "Received a startup command"
          }
        }
      }
      frame "Checking Vacuum" {
        n510 = stacked-sequence {
          seq-local: [w931 _] -> [_ w950]
          seq-local: [w930 _] -> [_ w949]
          seq-local: [w929 _] -> [_ w948]
          tunnel: w926 -> [_ w951]
          tunnel: [_ w952] -> w927
          frame #0 {
            n511 = Tick Count (ms)() -> (millisecond timer value=w932:u32)
            n512 = call "_FPGA Set LEDs.vi"("LED Command"=_LED_States."Off BRP") -> ("error out"=w928:errorcluster)  [unwired: 3 in, 3 out]
            n513 = while {
              tunnel: w932 -> [w944]
              tunnel: [w943] -> w931
              tunnel: [w941] -> w930
              tunnel: [w934] -> w929
              tunnel: w928 -> [_]
              stop <- w936 stop-if-true
              w938 = u32 1800000  # 30min timeout
              n514 = Wait (ms)(milliseconds to wait=u32 800) -> (millisecond timer value=w946:u32)
              n515 = Subtract(x=w946, y=w944) -> (x-y=w939:u32)
              n516 = call "_Check Limit.vi"("Header"="Pumping 2:" ("Header (10Ch)"), "Current"=w939, "Max (100)"=w938) -> ("Max Reached"=w937:bool, "ProgressBar"=w935:string)  [unwired: 1 in, 2 out]
              n517 = call "_FPGA Check Vacuum.vi"() -> ("Vac OK"=w943:bool, "Source OK"=w941:bool, "Stop"=w942:bool, "Shutdown"=w934:bool)  [unwired: 2 out]
              n518 = Or(x=w942, y=w937) -> (x .or. y?=w936:bool)
              n519 = case shown="False" w936 {
                tunnel: w935 -> [w947 _]
                frame False {
                  n520 = call "_FPGA Set LCD Msg.vi"("Info"=w947) -> ()  [unwired: 6 in, 3 out]
                }
                frame True {
                }
              }
            }
          }
          frame #1 {
            n521 = case shown="True" w950 {
              tunnel: [w955 w970] -> w952
              tunnel: w951 -> [_ w964]
              tunnel: w949 -> [_ w965]
              tunnel: w948 -> [w953 _]
              frame False {
                # "User aborted vacuum check or 20min timeout:\nHigh vacuum not achieved."
                n522 = case shown="False" w953 {
                  tunnel: [_RT_Instrument_State."Turbopump Ready" ("t") _RT_Instrument_State."Shutting Down" ("t")] -> w955
                  tunnel: [u8 1 ("StartupMode") u8 2 ("StartupMode")] -> w954
                  frame False {
                    w958 = T22 2 items=["Same", "Empty", "VacFail", "Cancel", "CheckGas", "EleFail", "Probe1Fail", "Probe2Fail", "HeaterFail", "DoorOpen", "CheckComm", "PressStart", "StartRP"] ("Line2Msg (same)")
                    w959 = T23 5 items=["Same", "Empty", "Connected", "Starting", "Stopping", "Action", "On", "Service", "Call", "Acquiring", "Source"] ("Line1Msg (same)")
                    n523 = call "_RT Event.vi"("Event"="Going to Turbopump Ready state.") -> ()  [unwired: 2 in, 5 out]
                    n524 = call "_FPGA Set LCD Msg.vi"("ErrNum"="003", "Line2Msg (same)"=w958, "Line1Msg (same)"=w959) -> ()  [unwired: 4 in, 3 out]
                  }
                  frame True {
                  }
                }
                n525 = global write "_RT Global.vi" "StartupMode"(w954) -> ()
              }
              frame True {
                # "High Vacuum Achieved"
                n526 = case shown="False" w965 {
                  tunnel: [_RT_Instrument_State."Source Standby" ("t") _RT_Instrument_State."Going to Ready" ("t")] -> w970
                  frame False {
                    n527 = call "_RT Event.vi"("Event"="Going to Source Standby state.") -> ()  [unwired: 2 in, 5 out]
                    n528 = global write "_RT Global.vi" "StartupMode"(u8 1 ("StartupMode")) -> ()
                  }
                  frame True {
                    # "Source OK"
                  }
                }
                n529 = xnode "Read/Write Control"("FPGA VI Reference In"=w964, "FilaB"=FALSE) -> ("FPGA VI Reference Out"=w967:refnum<k20>, "error out"=w968:errorcluster)  [unwired: 1 in]
                n530 = xnode "Read/Write Control"("FPGA VI Reference In"=w967, "error in"=w968, "FilaC"=TRUE) -> ()  [unwired: 2 out]
              }
            }
          }
        }
      }
      frame "Going to Ready" {
        w978 = T22 1 items=["Same", "Empty", "VacFail", "Cancel", "CheckGas", "EleFail", "Probe1Fail", "Probe2Fail", "HeaterFail", "DoorOpen", "CheckComm", "PressStart", "StartRP"] ("Line2Msg (same)")
        w979 = T23 6 items=["Same", "Empty", "Connected", "Starting", "Stopping", "Action", "On", "Service", "Call", "Acquiring", "Source"] ("Line1Msg (same)")
        n531 = call "_FPGA Set LEDs.vi"("LED Command"=_LED_States."Off BRP") -> ("error out"=w981:errorcluster)  [unwired: 3 in, 3 out]
        n532 = call "_FPGA Set LEDs.vi"("error in (no error)"=w981, "LED Command"=_LED_States."Solid P") -> ("error out"=w983:errorcluster)  [unwired: 2 in, 3 out]
        n533 = call "_FPGA Set LCD Msg.vi"("error in"=w983, "Line2Msg (same)"=w978, "Line1Msg (same)"=w979) -> ("error out"=w986:errorcluster)  [unwired: 4 in, 2 out]
        n534 = call "_RT Event.vi"("Event"="Analyzer is Ready") -> ()  [unwired: 2 in, 5 out]
        n535 = call "_FPGA Send LCD.vi"("error in (no error)"=w986, "Command"=_RT_LED_Num."ReadKey" ("LED#")) -> ("error out"=w975:errorcluster)  [unwired: 3 in, 3 out]
        n536 = call "_FPGA Set Parameters.vi"("error in"=w975, "Set Zero (on)"=FALSE) -> ()  [unwired: 7 in, 3 out]
        n537 = global write "_RT Global.vi" "StartupMode"(u8 0 ("StartupMode")) -> ()
        n538 = local write "Ready"(TRUE ("Status LED")) -> ()
        n539 = local write "Fault"(FALSE ("Status LED")) -> ()
      }
      frame "Ready", Default {
        n540 = local read "Connected?"() -> (w999:bool)
        n541 = call "_FPGA Read Key.vi"() -> ("error out"=w990:errorcluster, "Key Pressed"=w996:bool)  [unwired: 5 in, 2 out]
        n542 = local read "RunMode"() -> (w991:i32)
        n543 = call "_FPGA System Polling.vi"("error in (no error)"=w990, "Connected?"=w999, "CurInstrState"=w998) -> ("Running"=w992:bool, "Next InstrState"=w997:T2)  [unwired: 1 in, 3 out]
        n544 = case shown="3, 6, 7" w991 {
          tunnel: [_ TRUE] -> w995
          frame 0, Default {
          }
          frame 3, 6, 7 {
          }
        }
        n545 = local write "Running"(w992) -> ()
        n546 = And(x=w995, y=w992) -> (x .and. y?=w994:bool)
        n547 = case shown="True" w994 {
          tunnel: [w1002 _RT_Instrument_State."Running" ("InstrState")] -> w1000
          tunnel: w997 -> [w1010 _]
          tunnel: w996 -> [w1008 _]
          tunnel: w993 -> [w1005 w1018]
          tunnel: w992 -> [w1007 _]
          tunnel: w991 -> [w1006 _]
          frame False {
            n548 = Select(t=_RT_Instrument_State."Shutting Down", s=w1008, f=w1010) -> (s? t:f=w1002:T2)
            n549 = Not Equal?(x=w1002, y=_RT_Instrument_State."Ready" ("t")) -> (x != y?=w1004:bool)
            n550 = case shown="True" w1004 {
              tunnel: w1002 -> [_ w1014]
              tunnel: w1007 -> [_ w1013]
              tunnel: w1006 -> [_ w1012]
              tunnel: w1005 -> [_ w1011]
              frame False {
              }
              frame True {
                n551 = Format Into String(format string="Instr State transitioned from Ready to %s; FPGA Running = %s; Run Mode = %d; Loop = %d." ("Event"), w1014, w1013, w1012, w1011) -> (resulting string=w1015:string)  [unwired: 2 in, 1 out]
                n552 = call "_RT Event.vi"("Event"=w1015) -> ()  [unwired: 2 in, 5 out]
              }
            }
          }
          frame True {
            w1020 = T22 1 items=["Same", "Empty", "VacFail", "Cancel", "CheckGas", "EleFail", "Probe1Fail", "Probe2Fail", "HeaterFail", "DoorOpen", "CheckComm", "PressStart", "StartRP"] ("Line2Msg (same)")
            w1021 = T23 9 items=["Same", "Empty", "Connected", "Starting", "Stopping", "Action", "On", "Service", "Call", "Acquiring", "Source"] ("Line1Msg (same)")
            n553 = call "_FPGA Set LEDs.vi"("LED Command"=_LED_States."Solid B") -> ("error out"=w1022:errorcluster)  [unwired: 3 in, 3 out]
            n554 = Format Into String(format string="A run has started; Loop = %d." ("Event"), w1018) -> (resulting string=w1017:string)  [unwired: 2 in, 1 out]
            n555 = call "_FPGA Set LCD Msg.vi"("error in"=w1022, "Line2Msg (same)"=w1020, "Line1Msg (same)"=w1021) -> ()  [unwired: 4 in, 3 out]
            n556 = call "_RT Event.vi"("Event"=w1017) -> ()  [unwired: 2 in, 5 out]
          }
        }
      }
      frame "Source Standby" {
        n557 = global read "_RT Global.vi" "StartupMode"() -> (w1027:u8)
        n558 = case shown="Default" w1027 {
          tunnel: [w1037 _RT_Instrument_State."Shutting Down" ("InstrState") _RT_Instrument_State."Starting Up" ("InstrState")] -> w1026
          tunnel: w1025 -> [w1034 _ _]
          frame Default {
            # "Allow system to shut down from this state"
            n559 = local read "Connected?"() -> (w1036:bool)
            n560 = call "_FPGA Read Key.vi"("CurStartupMode (0)"=u8 1) -> ("error out"=w1030:errorcluster, "Key Pressed"=w1039:bool)  [unwired: 4 in, 2 out]
            n561 = call "_FPGA System Polling.vi"("error in (no error)"=w1030, "Waiting (F)"=TRUE, "Connected?"=w1036, "CurInstrState"=w1034) -> ("Running"=w1035:bool, "Next InstrState"=w1033:T2)  [unwired: 1 in, 2 out]
            n562 = local write "Running"(w1035) -> ()
            n563 = Select(t=_RT_Instrument_State."Shutting Down", s=w1039, f=w1033) -> (s? t:f=w1037:T2)
          }
          frame 2 {
            # "Received a shutdown command"
          }
          frame 0 {
            # "Received a startup command"
          }
        }
        n564 = local write "Fault"(TRUE ("Status LED")) -> ()
        n565 = local write "Ready"(FALSE ("Status LED")) -> ()
      }
      frame "Running" {
        n566 = local read "Connected?"() -> (w1043:bool)
        n567 = call "_FPGA System Polling.vi"("Connected?"=w1043, "CurInstrState"=w1044) -> ("Running"=w1045:bool, "Next InstrState"=w1046:T2)  [unwired: 3 in, 2 out]
        n568 = local write "Running"(w1045) -> ()
        n569 = case shown="False" w1045 {
          tunnel: [_RT_Instrument_State."Ready" ("InstrState") w1061] -> w1047
          tunnel: w1046 -> [_ w1061]
          tunnel: w1044 -> [_ w1063]
          tunnel: w1042 -> [_ _]
          frame False {
            w1048 = T22 1 items=["Same", "Empty", "VacFail", "Cancel", "CheckGas", "EleFail", "Probe1Fail", "Probe2Fail", "HeaterFail", "DoorOpen", "CheckComm", "PressStart", "StartRP"] ("Line2Msg (same)")
            w1049 = T23 6 items=["Same", "Empty", "Connected", "Starting", "Stopping", "Action", "On", "Service", "Call", "Acquiring", "Source"] ("Line1Msg (same)")
            n570 = call "_FPGA Set LEDs.vi"("LED Command"=_LED_States."Off BRP") -> ("error out"=w1050:errorcluster)  [unwired: 3 in, 3 out]
            n571 = local write "Fault"(FALSE ("Status LED")) -> ()
            n572 = call "_FPGA Set LEDs.vi"("error in (no error)"=w1050, "LED Command"=_LED_States."Solid P") -> ("error out"=w1052:errorcluster)  [unwired: 2 in, 3 out]
            n573 = local write "Ready"(TRUE ("Status LED")) -> ()
            n574 = call "_FPGA Set LCD Msg.vi"("error in"=w1052, "Line2Msg (same)"=w1048, "Line1Msg (same)"=w1049) -> ("error out"=w1053:errorcluster)  [unwired: 4 in, 2 out]
            n575 = call "_RT Event.vi"("Event"="A run ended normally, analyzer is ready") -> ()  [unwired: 2 in, 5 out]
            n576 = call "_FPGA Send LCD.vi"("error in (no error)"=w1053, "Command"=_RT_LED_Num."ReadKey" ("LED#")) -> ()  [unwired: 3 in, 4 out]
            n577 = global write "_RT Global.vi" "StartupMode"(u8 0 ("StartupMode")) -> ()
          }
          frame True {
            n578 = Not Equal?(x=w1063, y=w1061) -> (x != y?=w1062:bool)
            n579 = case shown="True" w1062 {
              tunnel: w1061 -> [_ w1067]
              frame False {
              }
              frame True {
                w1068 = u16 0 ("Address")
                # "End a Run"
                n580 = Format Into String(format string="A run unexpectedly ended as RT state changed from Running to %s.", w1067) -> (resulting string=w1065:string)  [unwired: 2 in, 1 out]
                n581 = call "_FPGA Set LEDs.vi"("LED Command"=_LED_States."Off B") -> ("error out"=w1064:errorcluster)  [unwired: 3 in, 3 out]
                n582 = call "_RT Event.vi"("Event"=w1065) -> ()  [unwired: 2 in, 5 out]
                n583 = call "_FPGA Write Data.vi"("error in"=w1064, "Data"=w1068, "Address"=w1068) -> ()  [unwired: 3 in, 3 out]
              }
            }
          }
        }
      }
      frame "Lost Communication" {
        # "Allow system to shutdown from this state"
        n584 = local read "Connected?"() -> (w1078:bool)
        n585 = call "_FPGA Read Key.vi"("CurStartupMode (0)"=u8 1) -> ("error out"=w1070:errorcluster, "Key Pressed"=w1072:bool)  [unwired: 4 in, 2 out]
        n586 = call "_FPGA System Polling.vi"("error in (no error)"=w1070, "Connected?"=w1078, "CurInstrState"=w1077) -> ("Running"=w1076:bool, "Next InstrState"=w1075:T2)  [unwired: 2 in, 2 out]
        n587 = local write "Running"(w1076) -> ()
        n588 = Select(t=_RT_Instrument_State."Shutting Down", s=w1072, f=w1075) -> (s? t:f=w1074:T2)
      }
      frame "Shutting Down" {
        n589 = global read "_RT Global.vi" "StartupMode"() -> (w1084:u8)
        n590 = local read "Fault"() -> (w1092:bool)
        n591 = Greater Than 0?(x=w1084) -> (x > 0?=w1089:bool)
        n592 = Or(x=w1092, y=w1089) -> (x .or. y?=w1091:bool)
        n593 = Equal?(x=w1084, y=u8 1) -> (x = y?=w1082:bool)
        n594 = Select(t="Going to Roughing Pump Ready" ("Event"), s=w1082, f="Stopping Analyzer" ("Event")) -> (s? t:f=w1079:string)
        n595 = call "_RT Event.vi"("Event"=w1079) -> ("error out"=w1087:errorcluster)  [unwired: 2 in, 4 out]
        n596 = call "_Update Shutting Down.vi"("error in (no error)"=w1087, "Fault"=w1091) -> ("error Out"=w1085:errorcluster, "InstrState"=w1088:T2)  [unwired: 1 in, 3 out]
        n597 = call "_FPGA Send LCD.vi"("error in (no error)"=w1085, "Command"=_RT_LED_Num."ReadKey" ("LED#")) -> ()  [unwired: 2 in, 5 out]
        n598 = local write "Ready"(FALSE ("Status LED")) -> ()
      }
      frame "Fault" {
        # "Level 1 failure found and perform a total shutdown"
        n599 = stacked-sequence {
          frame #0 {
            n600 = local write "Ready"(FALSE ("Status LED")) -> ()
            n601 = call "_FPGA Set LEDs.vi"("LED Command"=_LED_States."Solid R") -> ()  [unwired: 3 in, 4 out]
            n602 = local write "Fault"(TRUE ("Status LED")) -> ()
            n603 = Wait (ms)(milliseconds to wait=u32 1800) -> ()  [unwired: 1 out]
          }
          frame #1 {
            n604 = call "_FPGA Send LCD.vi"("Command"=_RT_LED_Num."ReadKey" ("LED#")) -> ()  [unwired: 4 in, 4 out]
            n605 = global write "_RT Global.vi" "StartupMode"(u8 2 ("StartupMode")) -> ()
          }
        }
      }
    }
    n606 = global write "_RT Global.vi" "InstrState"(w795) -> ()
    n607 = Wait (ms)(milliseconds to wait=u32 280) -> ()  [unwired: 1 out]
    "InstrState" <- w795
  }
  n608 = Get Date/Time In Seconds() -> (seconds since 1Jan1904=w17:timestamp)
  n609 = To Double Precision Float(number=w17) -> (double precision float=w2:dbl)
  n610 = while {
    tunnel: w2 -> [w1100]
    stop <- FALSE stop-if-true
    # "Control the User1 indicator"
    n611 = Get Date/Time In Seconds() -> (seconds since 1Jan1904=w1101:timestamp)
    n612 = To Double Precision Float(number=w1101) -> (double precision float=w1102:dbl)
    n613 = Subtract(x=w1102, y=w1100) -> (x-y=w1103:dbl)
    "Time (s)" <- w1103
    n614 = global write "_RT Global.vi" "RT Time(s)"(w1103) -> ()
    n615 = local read "Connected?"() -> (w1108:bool)
    n616 = Select(t=u32 1800 ("milliseconds to wait"), s=w1108, f=u32 280 ("milliseconds to wait")) -> (s? t:f=w1110:u32)
    n617 = call <vilib>:"RT LEDs.vi"("State"=3, "LED Num"=0) -> ()  [unwired: 4 in, 2 out]
    n618 = Wait (ms)(milliseconds to wait=w1110) -> ()  [unwired: 1 out]
  }
